vi "HandleObservationSync.vi"(8 "error in (no error)":errorcluster, 11 "S4ACS_GUI in":refnum<class "S4ACS_GUI.lvclass">) -> (0 "error out":errorcluster, 3 "S4ACS_GUI out":refnum<class "S4ACS_GUI.lvclass">)   [LabVIEW 2018, in "S4ACS_GUI.lvclass"]
uses:
  S4ACS_GUI.lvclass
  S4ACS_GUI.lvclass/S4ACS_GUI.ctl
  Instrument/Instrument.lvclass/Instrument.ctl
  Device/Optics/Optics.lvclass/Optics.ctl
  Server/Server.lvclass/Server.ctl
  Device/Optics/Opt_Selector/Opt_Selector.lvclass
  C:/Users/observer/Desktop/Sparc4GUI/SPARC4_GUI/Device/Optics/Optics.lvclass
  Acquisition/Acquisition.lvclass
  C:/Users/observer/Desktop/Sparc4GUI/SPARC4_GUI/Server/Server.lvclass
  SyncBox/Sync Box.lvclass
  Instrument/Instrument.lvclass
  StateMachine/State Machine.lvclass
  Trigger/Trigger.lvclass
  Channel/Channel.lvclass
  Device/Optics/Optics.lvclass
  Server/Server.lvclass
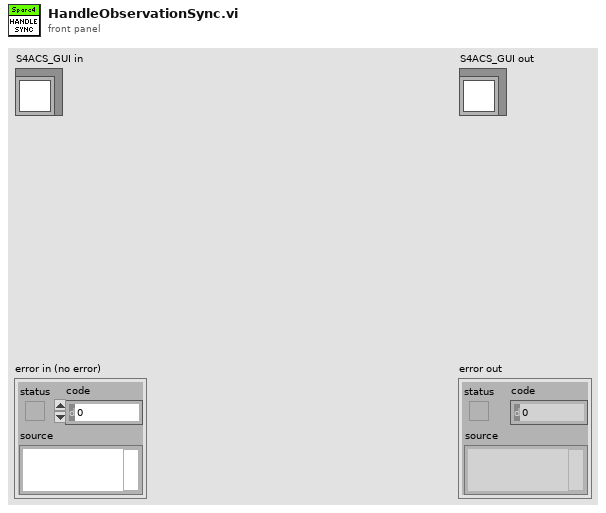
[diagram p1: front panel]
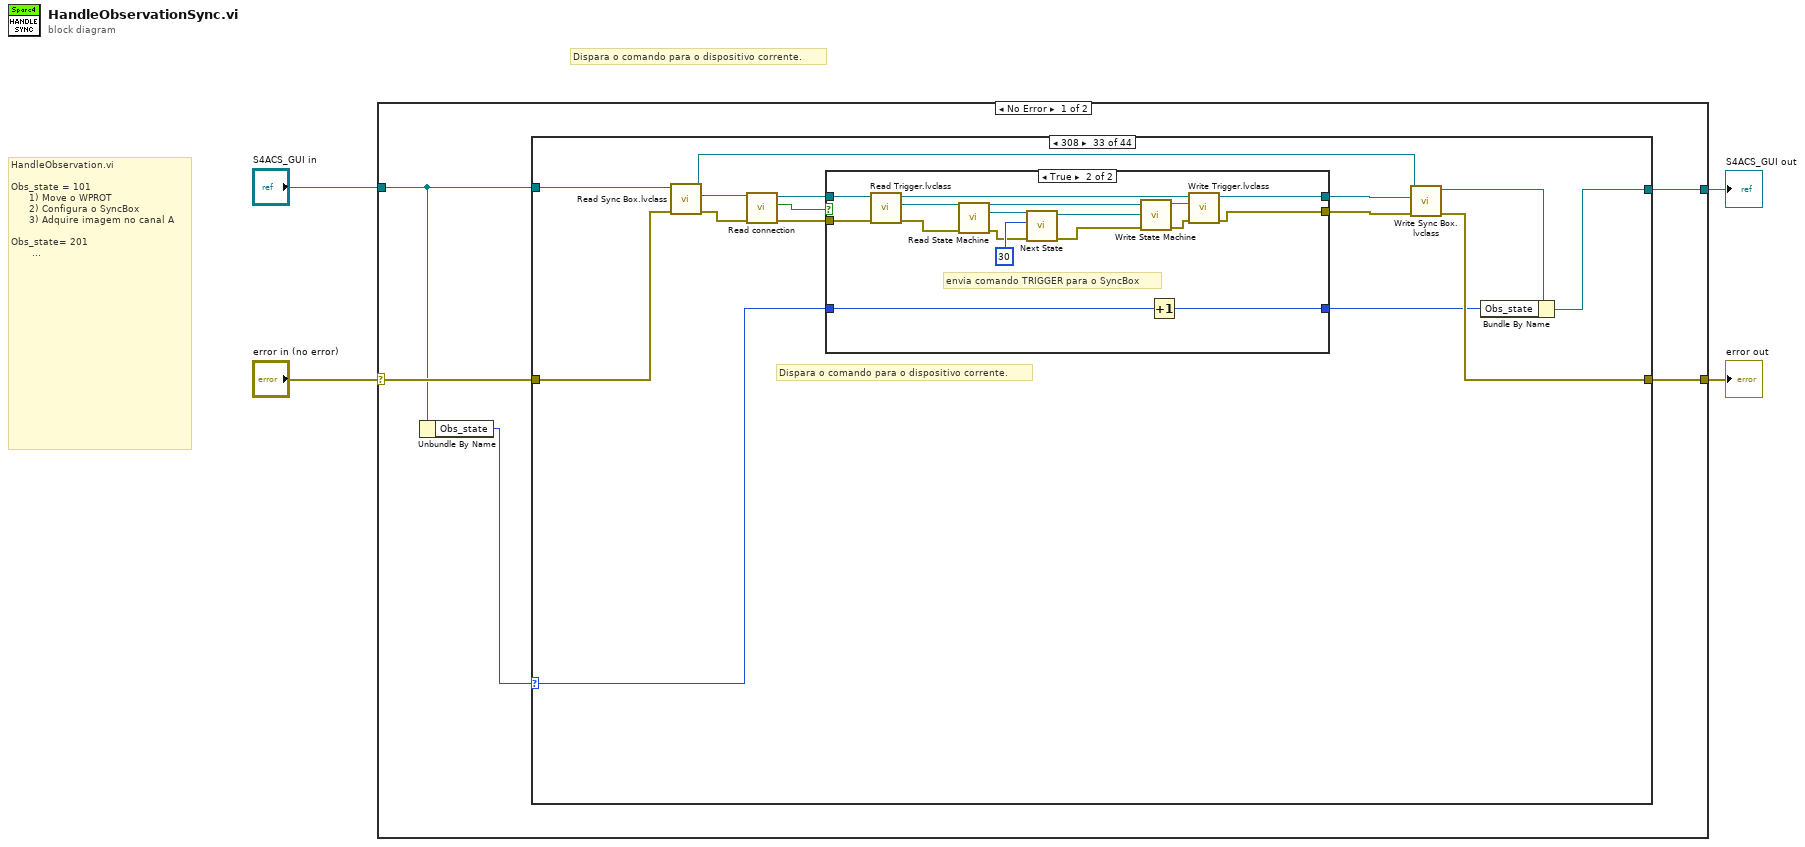
[diagram p0: block diagram]
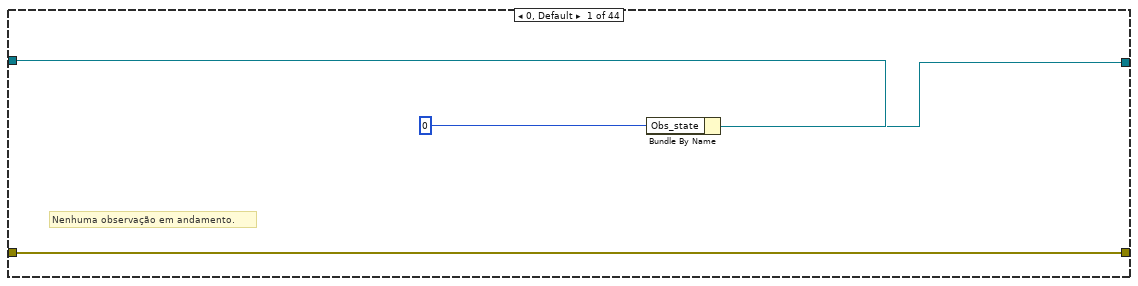
[diagram p2: hidden frame]
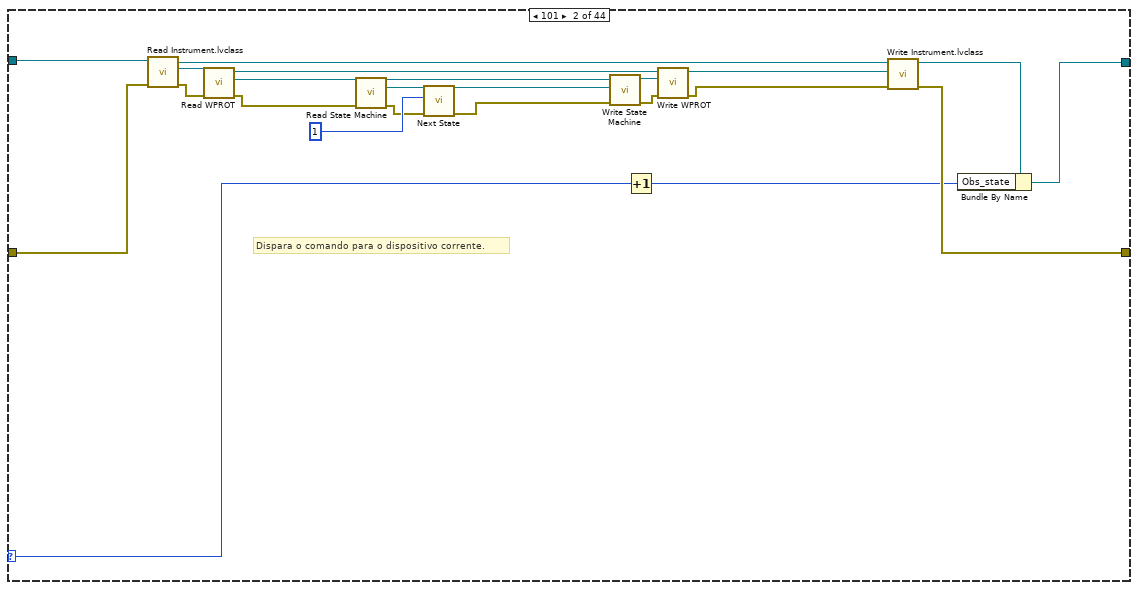
[diagram p3: hidden frame]
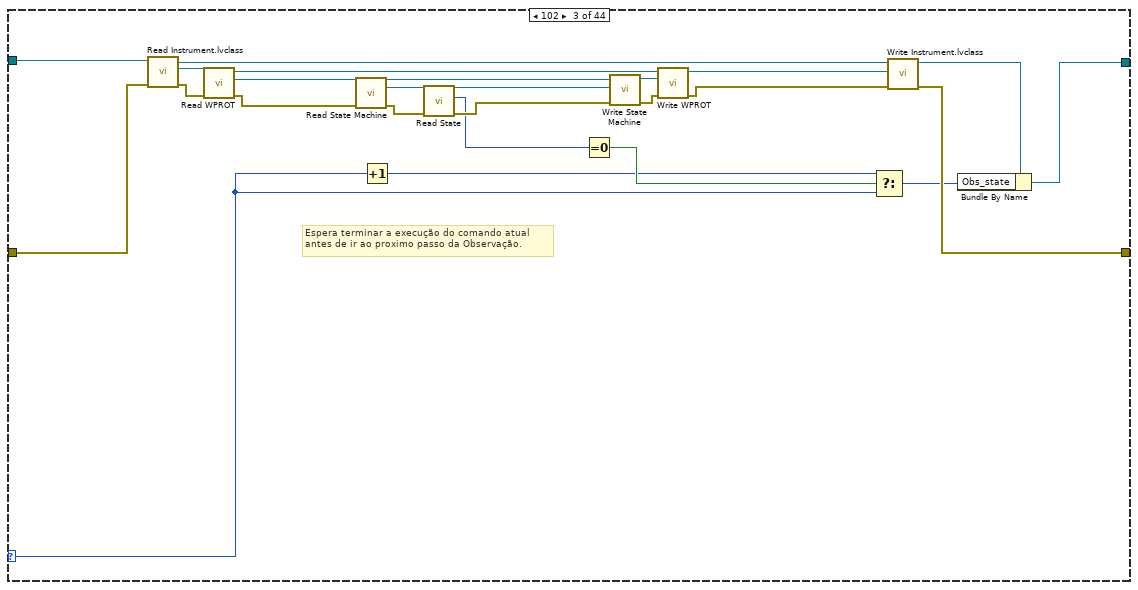
[diagram p4: hidden frame]
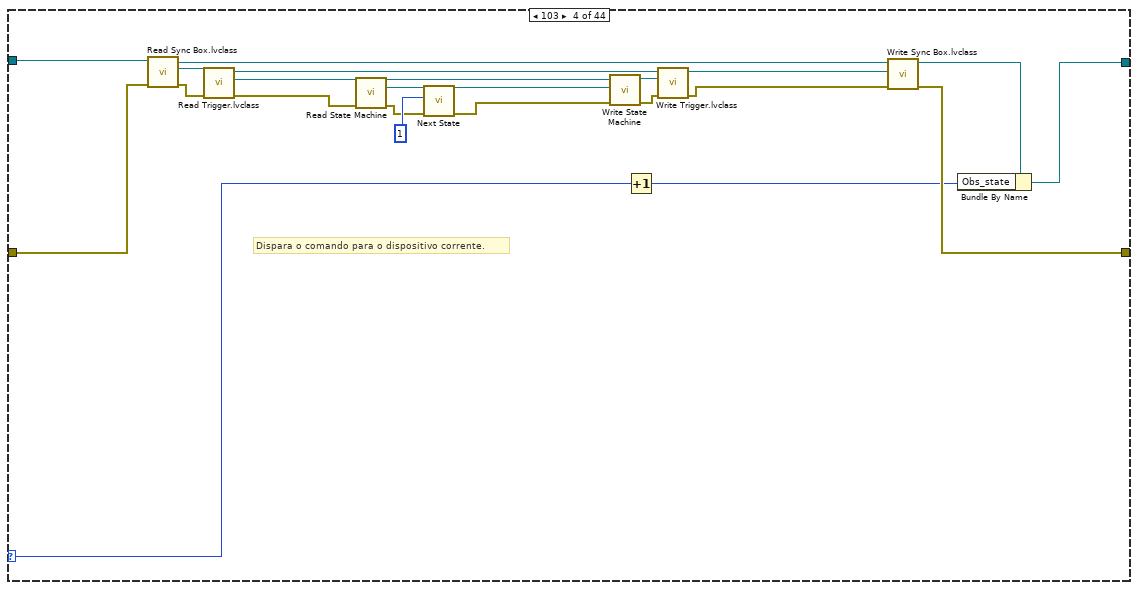
[diagram p5: hidden frame]
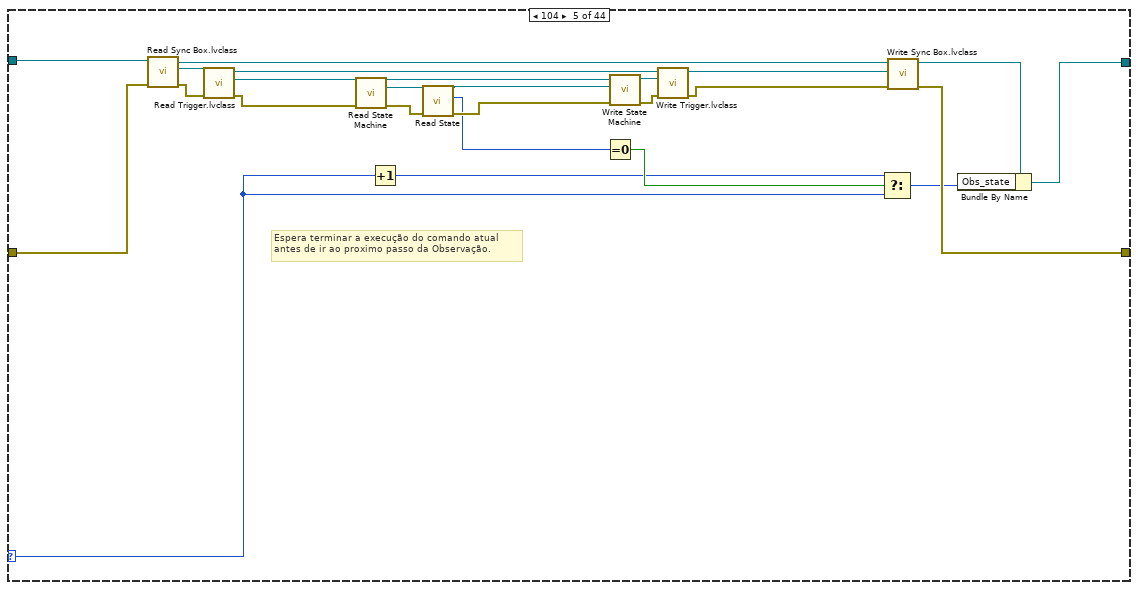
[diagram p6: hidden frame]
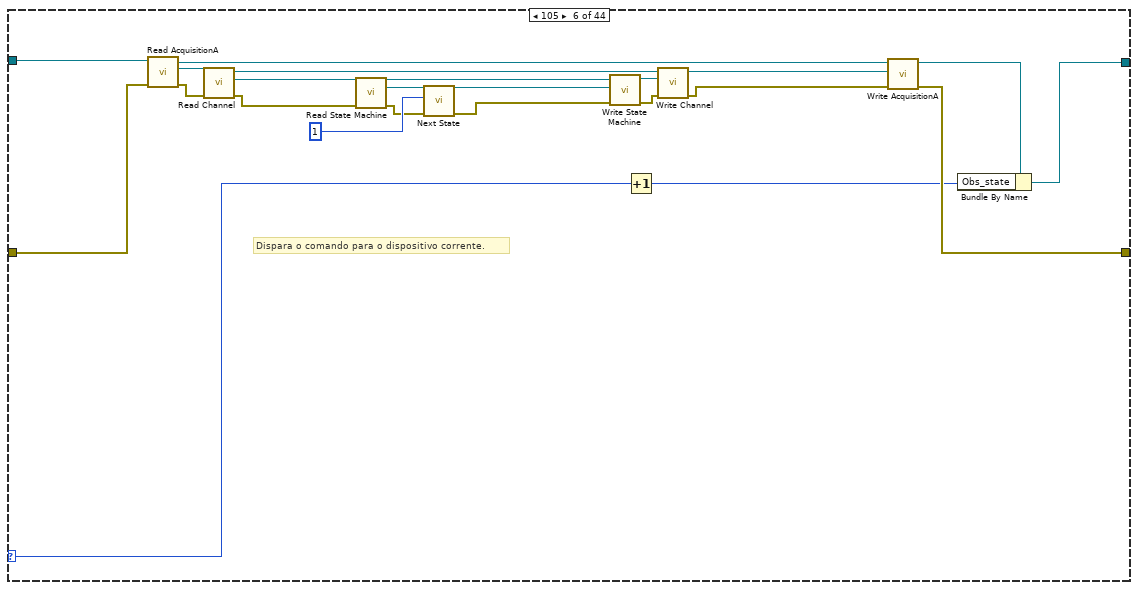
[diagram p7: hidden frame]
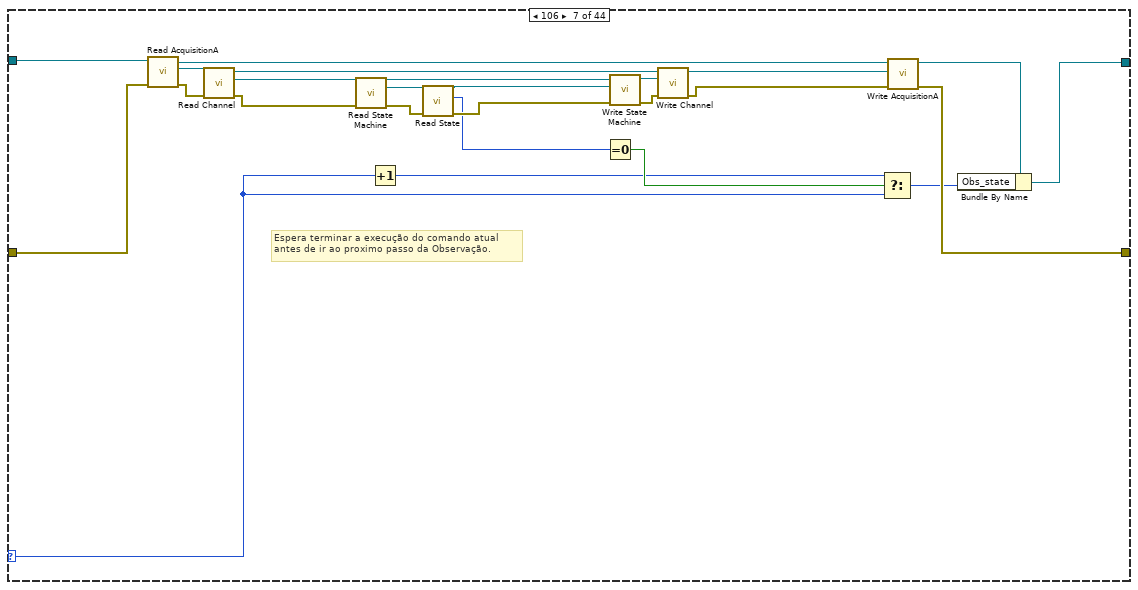
[diagram p8: hidden frame]
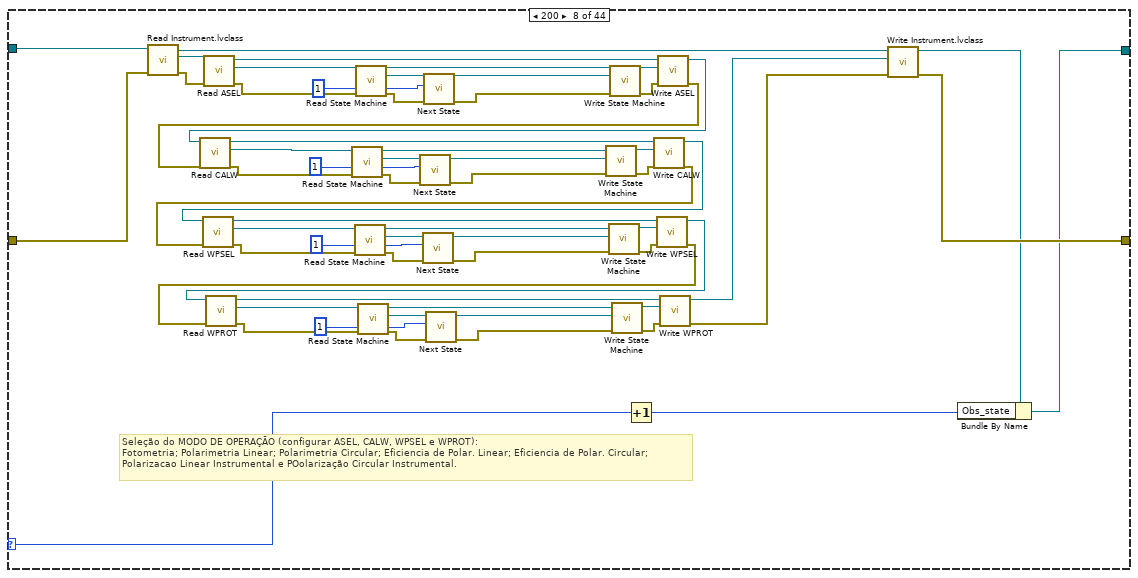
[diagram p9: hidden frame]
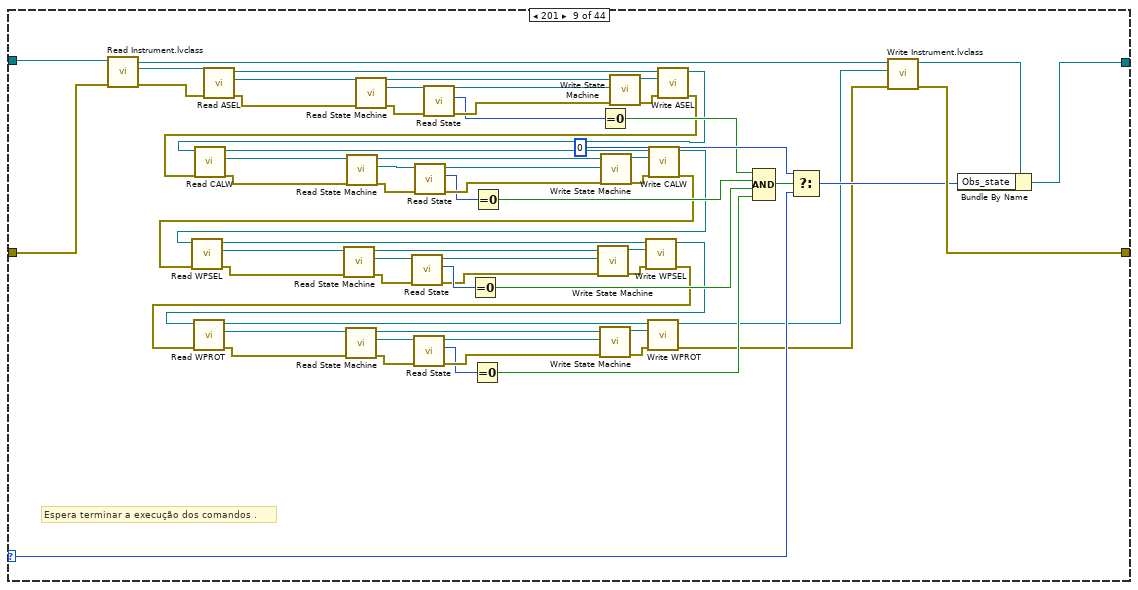
[diagram p10: hidden frame]
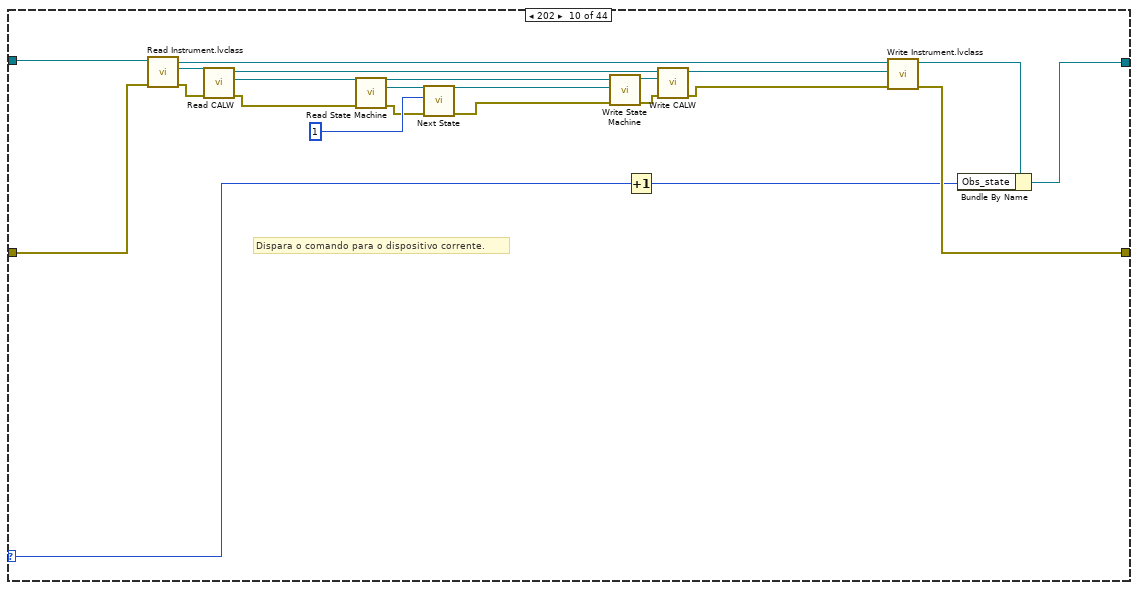
[diagram p11: hidden frame]
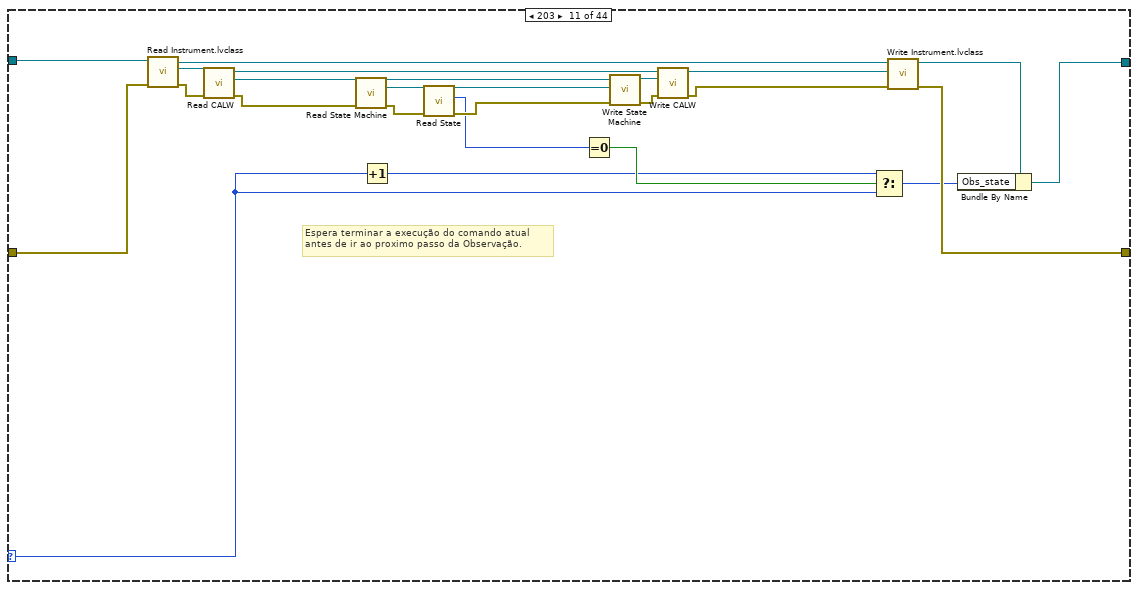
[diagram p12: hidden frame]
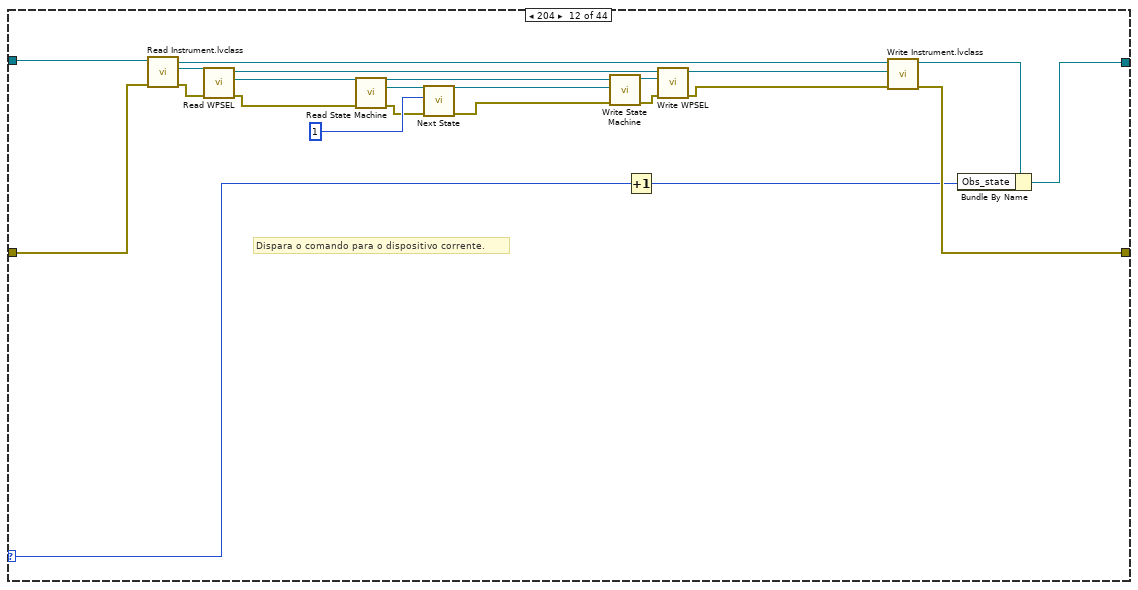
[diagram p13: hidden frame]
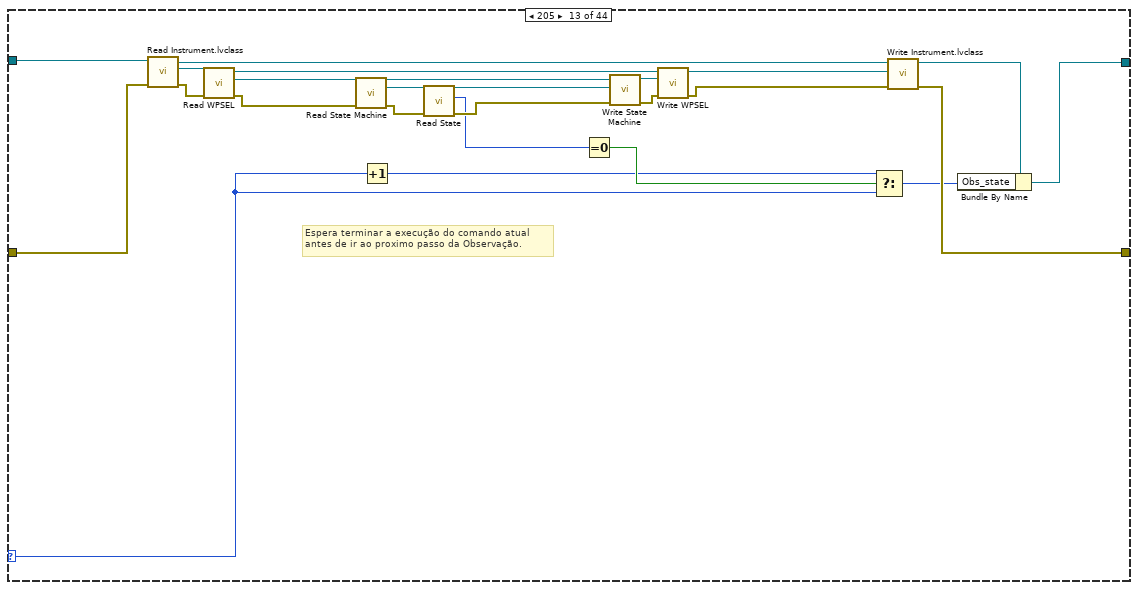
[diagram p14: hidden frame]
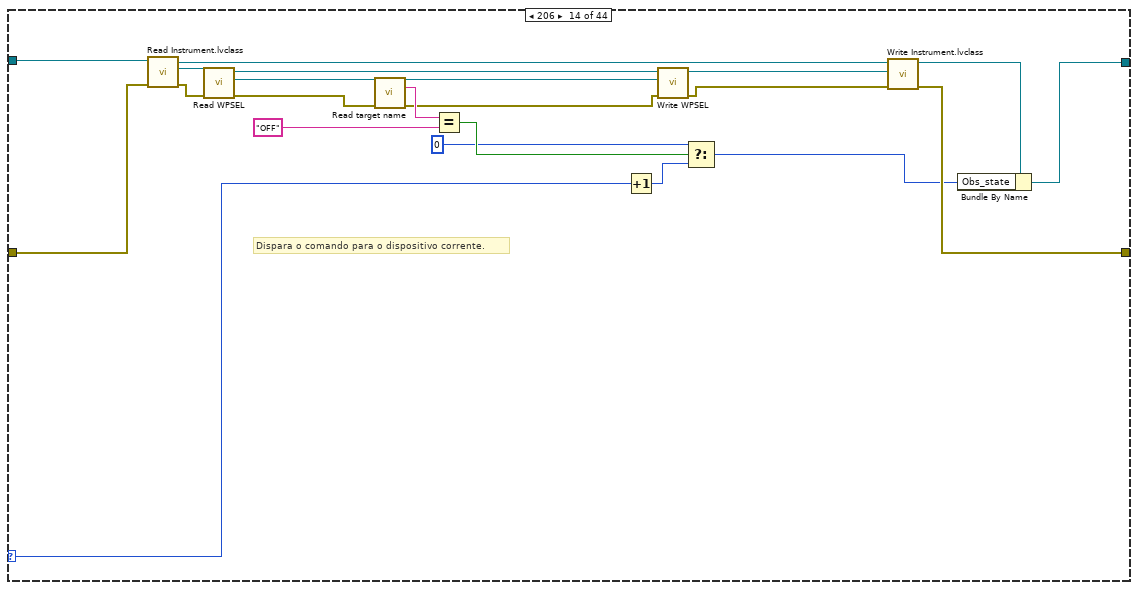
[diagram p15: hidden frame]
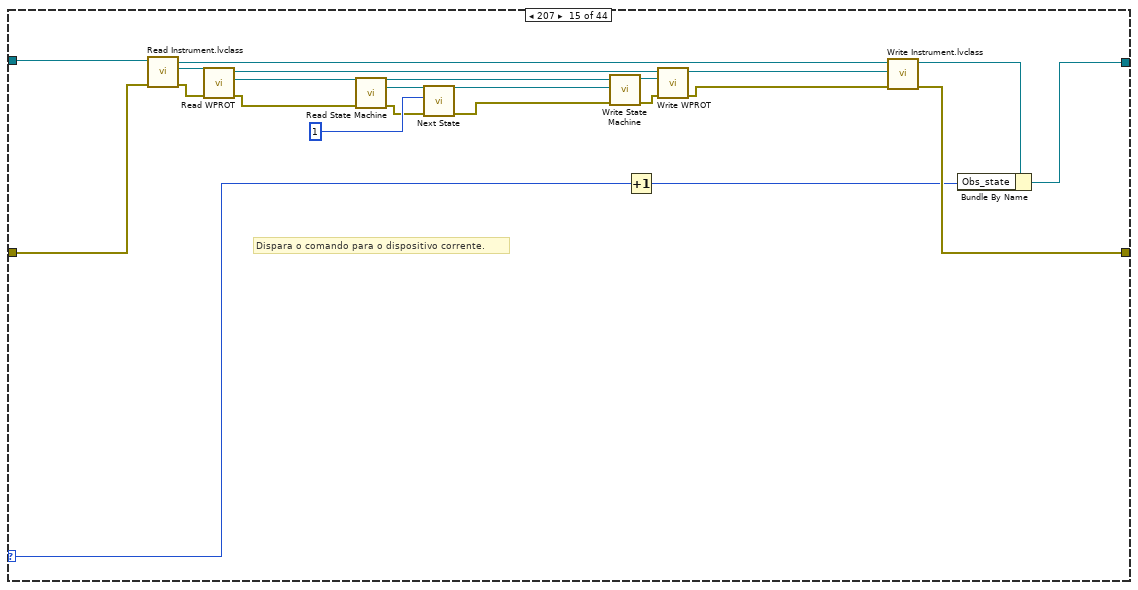
[diagram p16: hidden frame]
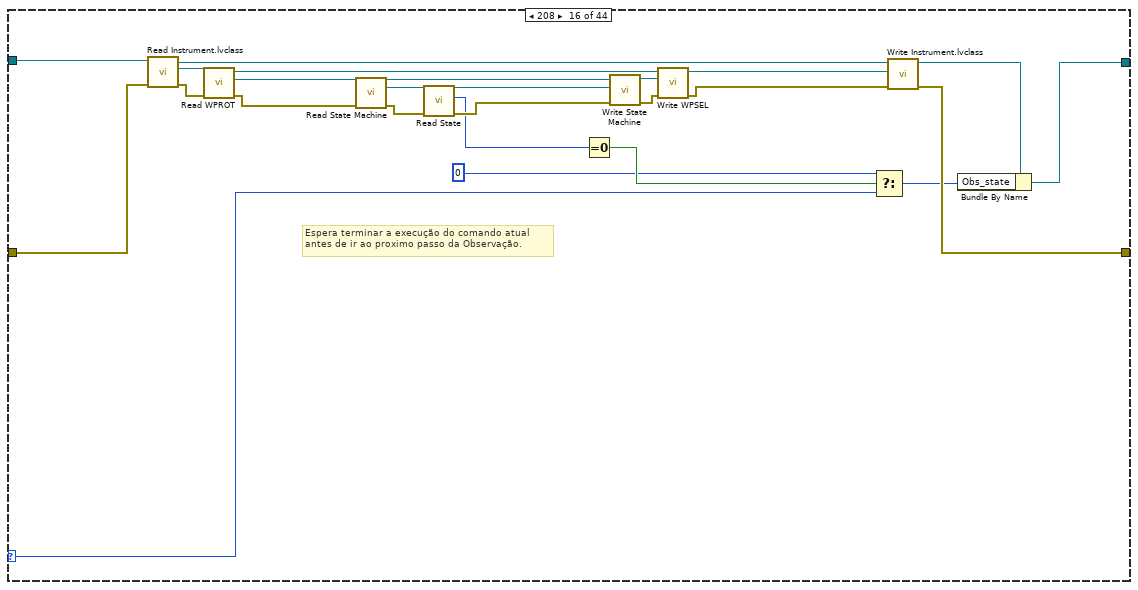
[diagram p17: hidden frame]
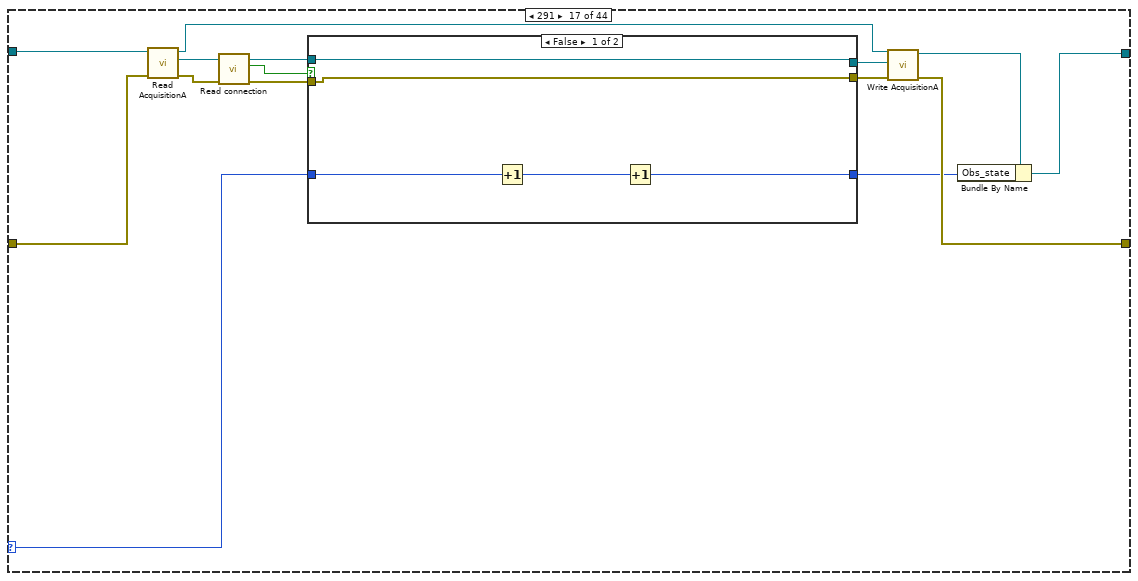
[diagram p18: hidden frame]
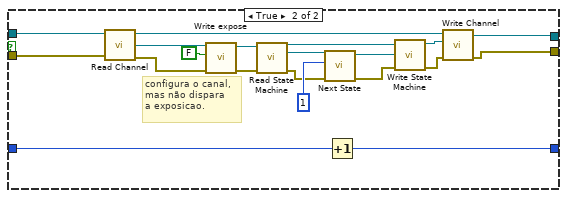
[diagram p19: hidden frame]
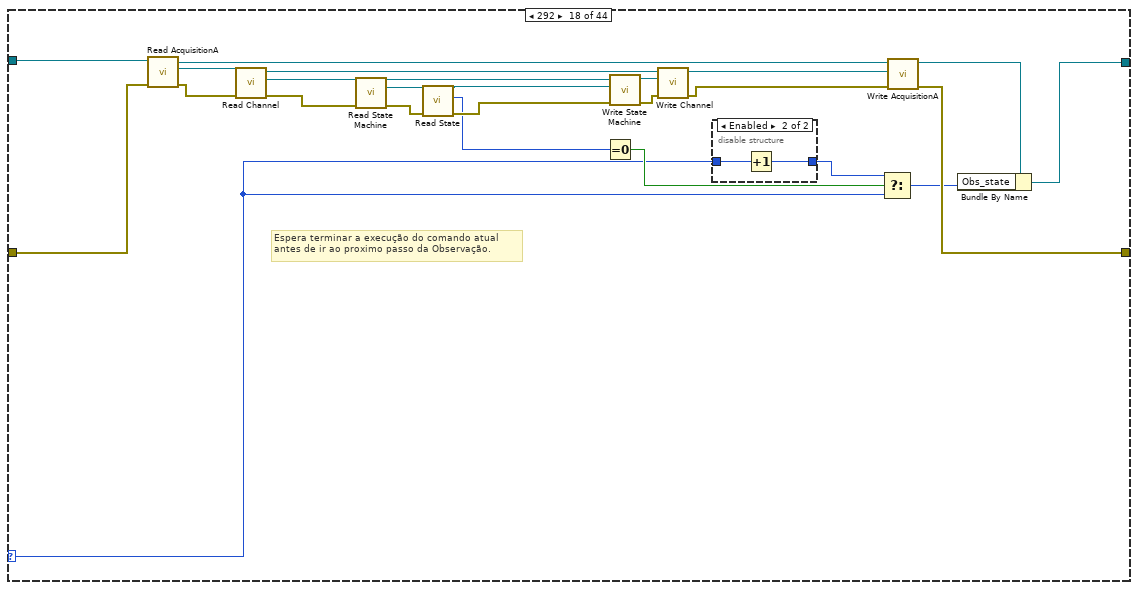
[diagram p20: hidden frame]
diagram:
  # "Dispara o comando para o dispositivo corrente."
  # "HandleObservation.vi\n\nObs_state = 101\n      1) Move o WPROT\n      2) Configura o SyncBox\n      3) Adquire imagem no canal A\n\nObs_state= 201\n       ..."
  n1 = case shown="No Error" "error in (no error)" {
    selector: "error in (no error)" -> [w8 w1585]
    tunnel: [w7 w1585] -> w3
    tunnel: [w9 w1584] -> w1
    tunnel: "S4ACS_GUI in" -> [w6 w1584]
    frame No Error {
      n2 = Unbundle By Name(w6) -> ("Obs_state"=w5:u32)
      n3 = case shown="308" w5 {
        selector: w5 -> [_ w16 w38 w64 w86 w112 w134 w202 w265 w290 w312 w338 w360 w395 w408 w430 w461 w494 w529 w563 w594 w628 w659 w693 _ w759 w805 w827 w858 w892 w955 w1041 w1077 w1108 w1187 _ w1232 w1272 w1340 w1422 w1459 w1543 _ _]
        tunnel: w6 -> [w12 w30 w55 w78 w103 w126 w151 w216 w283 w304 w329 w352 w377 w399 w422 w447 w465 w512 w533 w580 w598 w645 w663 w710 w727 w763 w820 w844 w862 w909 w957 w1058 w1081 w1125 w1205 w1225 w1242 w1289 w1299 w1432 w1476 w1556 w1576 w1583]
        tunnel: [w10 w14 w42 w62 w94 w110 w142 w200 w270 w288 w316 w336 w364 w394 w406 w434 w459 w503 w527 w571 w592 w636 w657 w701 w725 w757 w809 w835 w856 w900 w953 w1049 w1075 w1116 w1198 w1221 w1238 w1280 w1338 w1428 w1467 w1549 w1572 w1583] -> w9
        tunnel: w8 -> [w13 w29 w54 w77 w102 w125 w150 w215 w282 w303 w328 w351 w376 w398 w421 w446 w464 w511 w532 w579 w597 w644 w662 w709 w726 w762 w819 w843 w861 w908 w956 w1057 w1080 w1124 w1204 w1224 w1241 w1288 w1298 w1431 w1475 w1555 w1575 w1582]
        tunnel: [w13 w28 w53 w76 w101 w124 w149 w214 w281 w302 w327 w350 w375 w397 w420 w445 w463 w510 w531 w578 w596 w643 w661 w708 w717 w761 w818 w842 w860 w907 w937 w1056 w1079 w1123 w1132 w1223 w1240 w1287 w1296 w1430 w1474 w1485 w1574 w1582] -> w7
        frame 0, Default {
          # "Nenhuma observação em andamento."
          n4 = Bundle By Name(cluster=w12, "Obs_state"=u32 0) -> (w10:refnum<class "S4ACS_GUI.lvclass">)
        }
        frame 101 {
          # "Dispara o comando para o dispositivo corrente."
          n5 = call "Read Instrument.lvclass.vi"("error in (no error)"=w29, "S4ACS_GUI in"=w30) -> ("error out"=w35:errorcluster, "Instrument.lvclass"=w36:refnum<class "Instrument.lvclass">, "S4ACS_GUI out"=w32:refnum<class "S4ACS_GUI.lvclass">)  [unwired: 7 in]
          n6 = call "Read WPROT.vi"("error in (no error)"=w35, "Instrument in"=w36) -> ("error out"=w22:errorcluster, "Opt_Selector.lvclass"=w21:refnum<class "Opt_Selector.lvclass">, "Instrument out"=w34:refnum<class "Instrument.lvclass">)  [unwired: 7 in]
          n7 = call-dynamic "Read State Machine.vi"("error in (no error)"=w22, "Device in"=w21) -> ("error out"=w25:errorcluster, "State Machine.lvclass"=w27:refnum<class "State Machine.lvclass">, "Device out"=w19:refnum<class "Opt_Selector.lvclass">)  [unwired: 7 in]
          n8 = call "Next State.vi"("error in (no error)"=w25, "New_State"=1, "State Machine in"=w27) -> ("error out"=w24:errorcluster, "State Machine out"=w23:refnum<class "State Machine.lvclass">)  [unwired: 7 in]
          n9 = call-dynamic "Write State Machine.vi"("error in (no error)"=w24, "State Machine.lvclass"=w23, "Device in"=w19) -> ("error out"=w18:errorcluster, "Device out"=w20:refnum<class "Opt_Selector.lvclass">)  [unwired: 7 in]
          n10 = Increment(x=w16) -> (x+1=w15:u32)
          n11 = call "Write WPROT.vi"("error in (no error)"=w18, "Opt_Selector.lvclass"=w20, "Instrument in"=w34) -> ("error out"=w31:errorcluster, "Instrument out"=w33:refnum<class "Instrument.lvclass">)  [unwired: 7 in]
          n12 = call "Write Instrument.lvclass.vi"("error in (no error)"=w31, "Instrument.lvclass"=w33, "S4ACS_GUI in"=w32) -> ("error out"=w28:errorcluster, "S4ACS_GUI out"=w17:refnum<class "S4ACS_GUI.lvclass">)  [unwired: 7 in]
          n13 = Bundle By Name(cluster=w17, "Obs_state"=w15) -> (w14:refnum<class "S4ACS_GUI.lvclass">)
        }
        frame 102 {
          # "Espera terminar a execução do comando atual \nantes de ir ao proximo passo da Observação."
          n14 = call "Read Instrument.lvclass.vi"("error in (no error)"=w54, "S4ACS_GUI in"=w55) -> ("error out"=w60:errorcluster, "Instrument.lvclass"=w61:refnum<class "Instrument.lvclass">, "S4ACS_GUI out"=w57:refnum<class "S4ACS_GUI.lvclass">)  [unwired: 7 in]
          n15 = call "Read WPROT.vi"("error in (no error)"=w60, "Instrument in"=w61) -> ("error out"=w48:errorcluster, "Opt_Selector.lvclass"=w47:refnum<class "Opt_Selector.lvclass">, "Instrument out"=w59:refnum<class "Instrument.lvclass">)  [unwired: 7 in]
          n16 = call-dynamic "Read State Machine.vi"("error in (no error)"=w48, "Device in"=w47) -> ("error out"=w51:errorcluster, "State Machine.lvclass"=w52:refnum<class "State Machine.lvclass">, "Device out"=w45:refnum<class "Opt_Selector.lvclass">)  [unwired: 7 in]
          n17 = Increment(x=w38) -> (x+1=w37:u32)
          n18 = call-dynamic "Read State.vi"("error in (no error)"=w51, "State Machine in"=w52) -> ("error out"=w50:errorcluster, "State"=w40:i32, "State Machine out"=w49:refnum<class "State Machine.lvclass">)  [unwired: 7 in]
          n19 = Equal To 0?(x=w40) -> (x = 0?=w41:bool)
          n20 = call-dynamic "Write State Machine.vi"("error in (no error)"=w50, "State Machine.lvclass"=w49, "Device in"=w45) -> ("error out"=w44:errorcluster, "Device out"=w46:refnum<class "Opt_Selector.lvclass">)  [unwired: 7 in]
          n21 = call "Write WPROT.vi"("error in (no error)"=w44, "Opt_Selector.lvclass"=w46, "Instrument in"=w59) -> ("error out"=w56:errorcluster, "Instrument out"=w58:refnum<class "Instrument.lvclass">)  [unwired: 7 in]
          n22 = Select(t=w37, s=w41, f=w38) -> (s? t:f=w39:u32)
          n23 = call "Write Instrument.lvclass.vi"("error in (no error)"=w56, "Instrument.lvclass"=w58, "S4ACS_GUI in"=w57) -> ("error out"=w53:errorcluster, "S4ACS_GUI out"=w43:refnum<class "S4ACS_GUI.lvclass">)  [unwired: 7 in]
          n24 = Bundle By Name(cluster=w43, "Obs_state"=w39) -> (w42:refnum<class "S4ACS_GUI.lvclass">)
        }
        frame 103 {
          # "Dispara o comando para o dispositivo corrente."
          n25 = call-dynamic "Read Sync Box.lvclass.vi"("error in (no error)"=w77, "SPARC4_AC in"=w78) -> ("error out"=w83:errorcluster, "Sync Box.lvclass"=w84:refnum<class "Sync Box.lvclass">, "SPARC4_AC out"=w80:refnum<class "S4ACS_GUI.lvclass">)  [unwired: 7 in]
          n26 = call-dynamic "Read Trigger.lvclass.vi"("error in (no error)"=w83, "Sync Box in"=w84) -> ("error out"=w70:errorcluster, "Trigger.lvclass"=w69:refnum<class "Trigger.lvclass">, "Sync Box out"=w82:refnum<class "Sync Box.lvclass">)  [unwired: 7 in]
          n27 = call-dynamic "Read State Machine.vi"("error in (no error)"=w70, "Device in"=w69) -> ("error out"=w73:errorcluster, "State Machine.lvclass"=w75:refnum<class "State Machine.lvclass">, "Device out"=w67:refnum<class "Trigger.lvclass">)  [unwired: 7 in]
          n28 = call "Next State.vi"("error in (no error)"=w73, "New_State"=1, "State Machine in"=w75) -> ("error out"=w72:errorcluster, "State Machine out"=w71:refnum<class "State Machine.lvclass">)  [unwired: 7 in]
          n29 = call-dynamic "Write State Machine.vi"("error in (no error)"=w72, "State Machine.lvclass"=w71, "Device in"=w67) -> ("error out"=w66:errorcluster, "Device out"=w68:refnum<class "Trigger.lvclass">)  [unwired: 7 in]
          n30 = Increment(x=w64) -> (x+1=w63:u32)
          n31 = call-dynamic "Write Trigger.lvclass.vi"("error in (no error)"=w66, "Trigger.lvclass"=w68, "Sync Box in"=w82) -> ("error out"=w79:errorcluster, "Sync Box out"=w81:refnum<class "Sync Box.lvclass">)  [unwired: 7 in]
          n32 = call-dynamic "Write Sync Box.lvclass.vi"("error in (no error)"=w79, "Sync Box.lvclass"=w81, "SPARC4_AC in"=w80) -> ("error out"=w76:errorcluster, "SPARC4_AC out"=w65:refnum<class "S4ACS_GUI.lvclass">)  [unwired: 7 in]
          n33 = Bundle By Name(cluster=w65, "Obs_state"=w63) -> (w62:refnum<class "S4ACS_GUI.lvclass">)
        }
        frame 104 {
          # "Espera terminar a execução do comando atual \nantes de ir ao proximo passo da Observação."
          n34 = call-dynamic "Read Sync Box.lvclass.vi"("error in (no error)"=w102, "SPARC4_AC in"=w103) -> ("error out"=w108:errorcluster, "Sync Box.lvclass"=w109:refnum<class "Sync Box.lvclass">, "SPARC4_AC out"=w105:refnum<class "S4ACS_GUI.lvclass">)  [unwired: 7 in]
          n35 = call-dynamic "Read Trigger.lvclass.vi"("error in (no error)"=w108, "Sync Box in"=w109) -> ("error out"=w100:errorcluster, "Trigger.lvclass"=w99:refnum<class "Trigger.lvclass">, "Sync Box out"=w107:refnum<class "Sync Box.lvclass">)  [unwired: 7 in]
          n36 = call-dynamic "Read State Machine.vi"("error in (no error)"=w100, "Device in"=w99) -> ("error out"=w91:errorcluster, "State Machine.lvclass"=w93:refnum<class "State Machine.lvclass">, "Device out"=w97:refnum<class "Trigger.lvclass">)  [unwired: 7 in]
          n37 = Increment(x=w86) -> (x+1=w88:u32)
          n38 = call-dynamic "Read State.vi"("error in (no error)"=w91, "State Machine in"=w93) -> ("error out"=w90:errorcluster, "State"=w85:i32, "State Machine out"=w92:refnum<class "State Machine.lvclass">)  [unwired: 7 in]
          n39 = Equal To 0?(x=w85) -> (x = 0?=w89:bool)
          n40 = call-dynamic "Write State Machine.vi"("error in (no error)"=w90, "State Machine.lvclass"=w92, "Device in"=w97) -> ("error out"=w96:errorcluster, "Device out"=w98:refnum<class "Trigger.lvclass">)  [unwired: 7 in]
          n41 = call-dynamic "Write Trigger.lvclass.vi"("error in (no error)"=w96, "Trigger.lvclass"=w98, "Sync Box in"=w107) -> ("error out"=w104:errorcluster, "Sync Box out"=w106:refnum<class "Sync Box.lvclass">)  [unwired: 7 in]
          n42 = Select(t=w88, s=w89, f=w86) -> (s? t:f=w87:u32)
          n43 = call-dynamic "Write Sync Box.lvclass.vi"("error in (no error)"=w104, "Sync Box.lvclass"=w106, "SPARC4_AC in"=w105) -> ("error out"=w101:errorcluster, "SPARC4_AC out"=w95:refnum<class "S4ACS_GUI.lvclass">)  [unwired: 7 in]
          n44 = Bundle By Name(cluster=w95, "Obs_state"=w87) -> (w94:refnum<class "S4ACS_GUI.lvclass">)
        }
        frame 105 {
          # "Dispara o comando para o dispositivo corrente."
          n45 = call-dynamic "Read AcquisitionA.vi"("error in (no error)"=w125, "S4ACS_GUI in"=w126) -> ("error out"=w131:errorcluster, "Acquisition.lvclass"=w132:refnum<class "Acquisition.lvclass">, "S4ACS_GUI out"=w128:refnum<class "S4ACS_GUI.lvclass">)  [unwired: 7 in]
          n46 = call-dynamic "Read Channel.vi"("error in (no error)"=w131, "Acquisition in"=w132) -> ("error out"=w118:errorcluster, "Channel.lvclass"=w117:refnum<class "Channel.lvclass">, "Acquisition out"=w130:refnum<class "Acquisition.lvclass">)  [unwired: 7 in]
          n47 = call-dynamic "Read State Machine.vi"("error in (no error)"=w118, "Device in"=w117) -> ("error out"=w121:errorcluster, "State Machine.lvclass"=w123:refnum<class "State Machine.lvclass">, "Device out"=w115:refnum<class "Channel.lvclass">)  [unwired: 7 in]
          n48 = call "Next State.vi"("error in (no error)"=w121, "New_State"=1, "State Machine in"=w123) -> ("error out"=w120:errorcluster, "State Machine out"=w119:refnum<class "State Machine.lvclass">)  [unwired: 7 in]
          n49 = call-dynamic "Write State Machine.vi"("error in (no error)"=w120, "State Machine.lvclass"=w119, "Device in"=w115) -> ("error out"=w114:errorcluster, "Device out"=w116:refnum<class "Channel.lvclass">)  [unwired: 7 in]
          n50 = Increment(x=w112) -> (x+1=w111:u32)
          n51 = call-dynamic "Write Channel.vi"("error in (no error)"=w114, "Channel.lvclass"=w116, "Acquisition in"=w130) -> ("error out"=w127:errorcluster, "Acquisition out"=w129:refnum<class "Acquisition.lvclass">)  [unwired: 7 in]
          n52 = call-dynamic "Write AcquisitionA.vi"("error in (no error)"=w127, "Acquisition.lvclass"=w129, "S4ACS_GUI in"=w128) -> ("error out"=w124:errorcluster, "S4ACS_GUI out"=w113:refnum<class "S4ACS_GUI.lvclass">)  [unwired: 7 in]
          n53 = Bundle By Name(cluster=w113, "Obs_state"=w111) -> (w110:refnum<class "S4ACS_GUI.lvclass">)
        }
        frame 106 {
          # "Espera terminar a execução do comando atual \nantes de ir ao proximo passo da Observação."
          n54 = call-dynamic "Read AcquisitionA.vi"("error in (no error)"=w150, "S4ACS_GUI in"=w151) -> ("error out"=w156:errorcluster, "Acquisition.lvclass"=w157:refnum<class "Acquisition.lvclass">, "S4ACS_GUI out"=w153:refnum<class "S4ACS_GUI.lvclass">)  [unwired: 7 in]
          n55 = call-dynamic "Read Channel.vi"("error in (no error)"=w156, "Acquisition in"=w157) -> ("error out"=w148:errorcluster, "Channel.lvclass"=w147:refnum<class "Channel.lvclass">, "Acquisition out"=w155:refnum<class "Acquisition.lvclass">)  [unwired: 7 in]
          n56 = call-dynamic "Read State Machine.vi"("error in (no error)"=w148, "Device in"=w147) -> ("error out"=w139:errorcluster, "State Machine.lvclass"=w141:refnum<class "State Machine.lvclass">, "Device out"=w145:refnum<class "Channel.lvclass">)  [unwired: 7 in]
          n57 = Increment(x=w134) -> (x+1=w136:u32)
          n58 = call-dynamic "Read State.vi"("error in (no error)"=w139, "State Machine in"=w141) -> ("error out"=w138:errorcluster, "State"=w133:i32, "State Machine out"=w140:refnum<class "State Machine.lvclass">)  [unwired: 7 in]
          n59 = Equal To 0?(x=w133) -> (x = 0?=w137:bool)
          n60 = call-dynamic "Write State Machine.vi"("error in (no error)"=w138, "State Machine.lvclass"=w140, "Device in"=w145) -> ("error out"=w144:errorcluster, "Device out"=w146:refnum<class "Channel.lvclass">)  [unwired: 7 in]
          n61 = call-dynamic "Write Channel.vi"("error in (no error)"=w144, "Channel.lvclass"=w146, "Acquisition in"=w155) -> ("error out"=w152:errorcluster, "Acquisition out"=w154:refnum<class "Acquisition.lvclass">)  [unwired: 7 in]
          n62 = Select(t=w136, s=w137, f=w134) -> (s? t:f=w135:u32)
          n63 = call-dynamic "Write AcquisitionA.vi"("error in (no error)"=w152, "Acquisition.lvclass"=w154, "S4ACS_GUI in"=w153) -> ("error out"=w149:errorcluster, "S4ACS_GUI out"=w143:refnum<class "S4ACS_GUI.lvclass">)  [unwired: 7 in]
          n64 = Bundle By Name(cluster=w143, "Obs_state"=w135) -> (w142:refnum<class "S4ACS_GUI.lvclass">)
        }
        frame 200 {
          # "Seleção do MODO DE OPERAÇÃO (configurar ASEL, CALW, WPSEL e WPROT): \nFotometria; Polarimetria Linear; Polarimetria Circular; Eficiencia de Polar. Linear; Eficiencia de Polar. Circular;\nPolarizacao Linear Instrumental e POolarização Circular Instrumental."
          n65 = call "Read Instrument.lvclass.vi"("error in (no error)"=w215, "S4ACS_GUI in"=w216) -> ("error out"=w219:errorcluster, "Instrument.lvclass"=w179:refnum<class "Instrument.lvclass">, "S4ACS_GUI out"=w217:refnum<class "S4ACS_GUI.lvclass">)  [unwired: 7 in]
          n66 = call "Read ASEL.vi"("error in (no error)"=w219, "Instrument in"=w179) -> ("error out"=w208:errorcluster, "Opt_Selector.lvclass"=w207:refnum<class "Opt_Selector.lvclass">, "Instrument out"=w218:refnum<class "Instrument.lvclass">)  [unwired: 7 in]
          n67 = call-dynamic "Read State Machine.vi"("error in (no error)"=w208, "Device in"=w207) -> ("error out"=w211:errorcluster, "State Machine.lvclass"=w213:refnum<class "State Machine.lvclass">, "Device out"=w205:refnum<class "Opt_Selector.lvclass">)  [unwired: 7 in]
          n68 = call "Next State.vi"("error in (no error)"=w211, "New_State"=1, "State Machine in"=w213) -> ("error out"=w210:errorcluster, "State Machine out"=w209:refnum<class "State Machine.lvclass">)  [unwired: 7 in]
          n69 = call-dynamic "Write State Machine.vi"("error in (no error)"=w210, "State Machine.lvclass"=w209, "Device in"=w205) -> ("error out"=w204:errorcluster, "Device out"=w206:refnum<class "Opt_Selector.lvclass">)  [unwired: 7 in]
          n70 = Increment(x=w202) -> (x+1=w201:u32)
          n71 = call "Write ASEL.vi"("error in (no error)"=w204, "Opt_Selector.lvclass"=w206, "Instrument in"=w218) -> ("error out"=w160:errorcluster, "Instrument out"=w178:refnum<class "Instrument.lvclass">)  [unwired: 7 in]
          n72 = call "Read CALW.vi"("error in (no error)"=w160, "Instrument in"=w178) -> ("error out"=w195:errorcluster, "Opt_Selector.lvclass"=w196:refnum<class "Opt_Selector.lvclass">, "Instrument out"=w177:refnum<class "Instrument.lvclass">)  [unwired: 7 in]
          n73 = call-dynamic "Read State Machine.vi"("error in (no error)"=w195, "Device in"=w196) -> ("error out"=w192:errorcluster, "State Machine.lvclass"=w190:refnum<class "State Machine.lvclass">, "Device out"=w198:refnum<class "Opt_Selector.lvclass">)  [unwired: 7 in]
          n74 = call "Next State.vi"("error in (no error)"=w192, "New_State"=1, "State Machine in"=w190) -> ("error out"=w193:errorcluster, "State Machine out"=w194:refnum<class "State Machine.lvclass">)  [unwired: 7 in]
          n75 = call-dynamic "Write State Machine.vi"("error in (no error)"=w193, "State Machine.lvclass"=w194, "Device in"=w198) -> ("error out"=w199:errorcluster, "Device out"=w197:refnum<class "Opt_Selector.lvclass">)  [unwired: 7 in]
          n76 = call "Write CALW.vi"("error in (no error)"=w199, "Opt_Selector.lvclass"=w197, "Instrument in"=w177) -> ("error out"=w159:errorcluster, "Instrument out"=w176:refnum<class "Instrument.lvclass">)  [unwired: 7 in]
          n77 = call "Read WPSEL.vi"("error in (no error)"=w159, "Instrument in"=w176) -> ("error out"=w184:errorcluster, "Opt_Selector.lvclass"=w183:refnum<class "Opt_Selector.lvclass">, "Instrument out"=w175:refnum<class "Instrument.lvclass">)  [unwired: 7 in]
          n78 = call-dynamic "Read State Machine.vi"("error in (no error)"=w184, "Device in"=w183) -> ("error out"=w187:errorcluster, "State Machine.lvclass"=w189:refnum<class "State Machine.lvclass">, "Device out"=w181:refnum<class "Opt_Selector.lvclass">)  [unwired: 7 in]
          n79 = call "Next State.vi"("error in (no error)"=w187, "New_State"=1, "State Machine in"=w189) -> ("error out"=w186:errorcluster, "State Machine out"=w185:refnum<class "State Machine.lvclass">)  [unwired: 7 in]
          n80 = call-dynamic "Write State Machine.vi"("error in (no error)"=w186, "State Machine.lvclass"=w185, "Device in"=w181) -> ("error out"=w180:errorcluster, "Device out"=w182:refnum<class "Opt_Selector.lvclass">)  [unwired: 7 in]
          n81 = call "Write WPSEL.vi"("error in (no error)"=w180, "Opt_Selector.lvclass"=w182, "Instrument in"=w175) -> ("error out"=w158:errorcluster, "Instrument out"=w164:refnum<class "Instrument.lvclass">)  [unwired: 7 in]
          n82 = call "Read WPROT.vi"("error in (no error)"=w158, "Instrument in"=w164) -> ("error out"=w170:errorcluster, "Opt_Selector.lvclass"=w171:refnum<class "Opt_Selector.lvclass">, "Instrument out"=w163:refnum<class "Instrument.lvclass">)  [unwired: 7 in]
          n83 = call-dynamic "Read State Machine.vi"("error in (no error)"=w170, "Device in"=w171) -> ("error out"=w167:errorcluster, "State Machine.lvclass"=w165:refnum<class "State Machine.lvclass">, "Device out"=w173:refnum<class "Opt_Selector.lvclass">)  [unwired: 7 in]
          n84 = call "Next State.vi"("error in (no error)"=w167, "New_State"=1, "State Machine in"=w165) -> ("error out"=w168:errorcluster, "State Machine out"=w169:refnum<class "State Machine.lvclass">)  [unwired: 7 in]
          n85 = call-dynamic "Write State Machine.vi"("error in (no error)"=w168, "State Machine.lvclass"=w169, "Device in"=w173) -> ("error out"=w174:errorcluster, "Device out"=w172:refnum<class "Opt_Selector.lvclass">)  [unwired: 7 in]
          n86 = call "Write WPROT.vi"("error in (no error)"=w174, "Opt_Selector.lvclass"=w172, "Instrument in"=w163) -> ("error out"=w161:errorcluster, "Instrument out"=w162:refnum<class "Instrument.lvclass">)  [unwired: 7 in]
          n87 = call "Write Instrument.lvclass.vi"("error in (no error)"=w161, "Instrument.lvclass"=w162, "S4ACS_GUI in"=w217) -> ("error out"=w214:errorcluster, "S4ACS_GUI out"=w203:refnum<class "S4ACS_GUI.lvclass">)  [unwired: 7 in]
          n88 = Bundle By Name(cluster=w203, "Obs_state"=w201) -> (w200:refnum<class "S4ACS_GUI.lvclass">)
        }
        frame 201 {
          # "Espera terminar a execução dos comandos ."
          n89 = call "Read Instrument.lvclass.vi"("error in (no error)"=w282, "S4ACS_GUI in"=w283) -> ("error out"=w286:errorcluster, "Instrument.lvclass"=w287:refnum<class "Instrument.lvclass">, "S4ACS_GUI out"=w284:refnum<class "S4ACS_GUI.lvclass">)  [unwired: 7 in]
          n90 = call "Read ASEL.vi"("error in (no error)"=w286, "Instrument in"=w287) -> ("error out"=w276:errorcluster, "Opt_Selector.lvclass"=w275:refnum<class "Opt_Selector.lvclass">, "Instrument out"=w285:refnum<class "Instrument.lvclass">)  [unwired: 7 in]
          n91 = call-dynamic "Read State Machine.vi"("error in (no error)"=w276, "Device in"=w275) -> ("error out"=w279:errorcluster, "State Machine.lvclass"=w280:refnum<class "State Machine.lvclass">, "Device out"=w273:refnum<class "Opt_Selector.lvclass">)  [unwired: 7 in]
          n92 = call-dynamic "Read State.vi"("error in (no error)"=w279, "State Machine in"=w280) -> ("error out"=w278:errorcluster, "State"=w269:i32, "State Machine out"=w277:refnum<class "State Machine.lvclass">)  [unwired: 7 in]
          n93 = Equal To 0?(x=w269) -> (x = 0?=w264:bool)
          n94 = call-dynamic "Write State Machine.vi"("error in (no error)"=w278, "State Machine.lvclass"=w277, "Device in"=w273) -> ("error out"=w272:errorcluster, "Device out"=w274:refnum<class "Opt_Selector.lvclass">)  [unwired: 7 in]
          n95 = call "Write ASEL.vi"("error in (no error)"=w272, "Opt_Selector.lvclass"=w274, "Instrument in"=w285) -> ("error out"=w226:errorcluster, "Instrument out"=w227:refnum<class "Instrument.lvclass">)  [unwired: 7 in]
          n96 = call "Read CALW.vi"("error in (no error)"=w226, "Instrument in"=w227) -> ("error out"=w259:errorcluster, "Opt_Selector.lvclass"=w260:refnum<class "Opt_Selector.lvclass">, "Instrument out"=w230:refnum<class "Instrument.lvclass">)  [unwired: 7 in]
          n97 = call-dynamic "Read State Machine.vi"("error in (no error)"=w259, "Device in"=w260) -> ("error out"=w256:errorcluster, "State Machine.lvclass"=w255:refnum<class "State Machine.lvclass">, "Device out"=w262:refnum<class "Opt_Selector.lvclass">)  [unwired: 7 in]
          n98 = call-dynamic "Read State.vi"("error in (no error)"=w256, "State Machine in"=w255) -> ("error out"=w257:errorcluster, "State"=w254:i32, "State Machine out"=w258:refnum<class "State Machine.lvclass">)  [unwired: 7 in]
          n99 = Equal To 0?(x=w254) -> (x = 0?=w253:bool)
          n100 = call-dynamic "Write State Machine.vi"("error in (no error)"=w257, "State Machine.lvclass"=w258, "Device in"=w262) -> ("error out"=w263:errorcluster, "Device out"=w261:refnum<class "Opt_Selector.lvclass">)  [unwired: 7 in]
          n101 = call "Write CALW.vi"("error in (no error)"=w263, "Opt_Selector.lvclass"=w261, "Instrument in"=w230) -> ("error out"=w224:errorcluster, "Instrument out"=w225:refnum<class "Instrument.lvclass">)  [unwired: 7 in]
          n102 = call "Read WPSEL.vi"("error in (no error)"=w224, "Instrument in"=w225) -> ("error out"=w247:errorcluster, "Opt_Selector.lvclass"=w246:refnum<class "Opt_Selector.lvclass">, "Instrument out"=w229:refnum<class "Instrument.lvclass">)  [unwired: 7 in]
          n103 = call-dynamic "Read State Machine.vi"("error in (no error)"=w247, "Device in"=w246) -> ("error out"=w250:errorcluster, "State Machine.lvclass"=w251:refnum<class "State Machine.lvclass">, "Device out"=w244:refnum<class "Opt_Selector.lvclass">)  [unwired: 7 in]
          n104 = call-dynamic "Read State.vi"("error in (no error)"=w250, "State Machine in"=w251) -> ("error out"=w249:errorcluster, "State"=w252:i32, "State Machine out"=w248:refnum<class "State Machine.lvclass">)  [unwired: 7 in]
          n105 = Equal To 0?(x=w252) -> (x = 0?=w232:bool)
          n106 = call-dynamic "Write State Machine.vi"("error in (no error)"=w249, "State Machine.lvclass"=w248, "Device in"=w244) -> ("error out"=w243:errorcluster, "Device out"=w245:refnum<class "Opt_Selector.lvclass">)  [unwired: 7 in]
          n107 = call "Write WPSEL.vi"("error in (no error)"=w243, "Opt_Selector.lvclass"=w245, "Instrument in"=w229) -> ("error out"=w222:errorcluster, "Instrument out"=w223:refnum<class "Instrument.lvclass">)  [unwired: 7 in]
          n108 = call "Read WPROT.vi"("error in (no error)"=w222, "Instrument in"=w223) -> ("error out"=w238:errorcluster, "Opt_Selector.lvclass"=w239:refnum<class "Opt_Selector.lvclass">, "Instrument out"=w228:refnum<class "Instrument.lvclass">)  [unwired: 7 in]
          n109 = call-dynamic "Read State Machine.vi"("error in (no error)"=w238, "Device in"=w239) -> ("error out"=w235:errorcluster, "State Machine.lvclass"=w234:refnum<class "State Machine.lvclass">, "Device out"=w241:refnum<class "Opt_Selector.lvclass">)  [unwired: 7 in]
          n110 = call-dynamic "Read State.vi"("error in (no error)"=w235, "State Machine in"=w234) -> ("error out"=w236:errorcluster, "State"=w233:i32, "State Machine out"=w237:refnum<class "State Machine.lvclass">)  [unwired: 7 in]
          n111 = Equal To 0?(x=w233) -> (x = 0?=w231:bool)
          n112 = call-dynamic "Write State Machine.vi"("error in (no error)"=w236, "State Machine.lvclass"=w237, "Device in"=w241) -> ("error out"=w242:errorcluster, "Device out"=w240:refnum<class "Opt_Selector.lvclass">)  [unwired: 7 in]
          n113 = call "Write WPROT.vi"("error in (no error)"=w242, "Opt_Selector.lvclass"=w240, "Instrument in"=w228) -> ("error out"=w220:errorcluster, "Instrument out"=w221:refnum<class "Instrument.lvclass">)  [unwired: 7 in]
          n114 = Compound Arithmetic op=AND(w264, w253, w232, w231) -> (w266:bool)
          n115 = Select(t=u32 0, s=w266, f=w265) -> (s? t:f=w268:u32)
          n116 = call "Write Instrument.lvclass.vi"("error in (no error)"=w220, "Instrument.lvclass"=w221, "S4ACS_GUI in"=w284) -> ("error out"=w281:errorcluster, "S4ACS_GUI out"=w271:refnum<class "S4ACS_GUI.lvclass">)  [unwired: 7 in]
          n117 = Bundle By Name(cluster=w271, "Obs_state"=w268) -> (w270:refnum<class "S4ACS_GUI.lvclass">)
        }
        frame 202 {
          # "Dispara o comando para o dispositivo corrente."
          n118 = call "Read Instrument.lvclass.vi"("error in (no error)"=w303, "S4ACS_GUI in"=w304) -> ("error out"=w309:errorcluster, "Instrument.lvclass"=w310:refnum<class "Instrument.lvclass">, "S4ACS_GUI out"=w306:refnum<class "S4ACS_GUI.lvclass">)  [unwired: 7 in]
          n119 = call "Read CALW.vi"("error in (no error)"=w309, "Instrument in"=w310) -> ("error out"=w296:errorcluster, "Opt_Selector.lvclass"=w295:refnum<class "Opt_Selector.lvclass">, "Instrument out"=w308:refnum<class "Instrument.lvclass">)  [unwired: 7 in]
          n120 = call-dynamic "Read State Machine.vi"("error in (no error)"=w296, "Device in"=w295) -> ("error out"=w299:errorcluster, "State Machine.lvclass"=w301:refnum<class "State Machine.lvclass">, "Device out"=w293:refnum<class "Opt_Selector.lvclass">)  [unwired: 7 in]
          n121 = call "Next State.vi"("error in (no error)"=w299, "New_State"=1, "State Machine in"=w301) -> ("error out"=w298:errorcluster, "State Machine out"=w297:refnum<class "State Machine.lvclass">)  [unwired: 7 in]
          n122 = call-dynamic "Write State Machine.vi"("error in (no error)"=w298, "State Machine.lvclass"=w297, "Device in"=w293) -> ("error out"=w292:errorcluster, "Device out"=w294:refnum<class "Opt_Selector.lvclass">)  [unwired: 7 in]
          n123 = Increment(x=w290) -> (x+1=w289:u32)
          n124 = call "Write CALW.vi"("error in (no error)"=w292, "Opt_Selector.lvclass"=w294, "Instrument in"=w308) -> ("error out"=w305:errorcluster, "Instrument out"=w307:refnum<class "Instrument.lvclass">)  [unwired: 7 in]
          n125 = call "Write Instrument.lvclass.vi"("error in (no error)"=w305, "Instrument.lvclass"=w307, "S4ACS_GUI in"=w306) -> ("error out"=w302:errorcluster, "S4ACS_GUI out"=w291:refnum<class "S4ACS_GUI.lvclass">)  [unwired: 7 in]
          n126 = Bundle By Name(cluster=w291, "Obs_state"=w289) -> (w288:refnum<class "S4ACS_GUI.lvclass">)
        }
        frame 203 {
          # "Espera terminar a execução do comando atual \nantes de ir ao proximo passo da Observação."
          n127 = call "Read Instrument.lvclass.vi"("error in (no error)"=w328, "S4ACS_GUI in"=w329) -> ("error out"=w334:errorcluster, "Instrument.lvclass"=w335:refnum<class "Instrument.lvclass">, "S4ACS_GUI out"=w331:refnum<class "S4ACS_GUI.lvclass">)  [unwired: 7 in]
          n128 = call "Read CALW.vi"("error in (no error)"=w334, "Instrument in"=w335) -> ("error out"=w322:errorcluster, "Opt_Selector.lvclass"=w321:refnum<class "Opt_Selector.lvclass">, "Instrument out"=w333:refnum<class "Instrument.lvclass">)  [unwired: 7 in]
          n129 = call-dynamic "Read State Machine.vi"("error in (no error)"=w322, "Device in"=w321) -> ("error out"=w325:errorcluster, "State Machine.lvclass"=w326:refnum<class "State Machine.lvclass">, "Device out"=w319:refnum<class "Opt_Selector.lvclass">)  [unwired: 7 in]
          n130 = Increment(x=w312) -> (x+1=w311:u32)
          n131 = call-dynamic "Read State.vi"("error in (no error)"=w325, "State Machine in"=w326) -> ("error out"=w324:errorcluster, "State"=w314:i32, "State Machine out"=w323:refnum<class "State Machine.lvclass">)  [unwired: 7 in]
          n132 = Equal To 0?(x=w314) -> (x = 0?=w315:bool)
          n133 = call-dynamic "Write State Machine.vi"("error in (no error)"=w324, "State Machine.lvclass"=w323, "Device in"=w319) -> ("error out"=w318:errorcluster, "Device out"=w320:refnum<class "Opt_Selector.lvclass">)  [unwired: 7 in]
          n134 = call "Write CALW.vi"("error in (no error)"=w318, "Opt_Selector.lvclass"=w320, "Instrument in"=w333) -> ("error out"=w330:errorcluster, "Instrument out"=w332:refnum<class "Instrument.lvclass">)  [unwired: 7 in]
          n135 = Select(t=w311, s=w315, f=w312) -> (s? t:f=w313:u32)
          n136 = call "Write Instrument.lvclass.vi"("error in (no error)"=w330, "Instrument.lvclass"=w332, "S4ACS_GUI in"=w331) -> ("error out"=w327:errorcluster, "S4ACS_GUI out"=w317:refnum<class "S4ACS_GUI.lvclass">)  [unwired: 7 in]
          n137 = Bundle By Name(cluster=w317, "Obs_state"=w313) -> (w316:refnum<class "S4ACS_GUI.lvclass">)
        }
        frame 204 {
          # "Dispara o comando para o dispositivo corrente."
          n138 = call "Read Instrument.lvclass.vi"("error in (no error)"=w351, "S4ACS_GUI in"=w352) -> ("error out"=w357:errorcluster, "Instrument.lvclass"=w358:refnum<class "Instrument.lvclass">, "S4ACS_GUI out"=w354:refnum<class "S4ACS_GUI.lvclass">)  [unwired: 7 in]
          n139 = call "Read WPSEL.vi"("error in (no error)"=w357, "Instrument in"=w358) -> ("error out"=w344:errorcluster, "Opt_Selector.lvclass"=w343:refnum<class "Opt_Selector.lvclass">, "Instrument out"=w356:refnum<class "Instrument.lvclass">)  [unwired: 7 in]
          n140 = call-dynamic "Read State Machine.vi"("error in (no error)"=w344, "Device in"=w343) -> ("error out"=w347:errorcluster, "State Machine.lvclass"=w349:refnum<class "State Machine.lvclass">, "Device out"=w341:refnum<class "Opt_Selector.lvclass">)  [unwired: 7 in]
          n141 = call "Next State.vi"("error in (no error)"=w347, "New_State"=1, "State Machine in"=w349) -> ("error out"=w346:errorcluster, "State Machine out"=w345:refnum<class "State Machine.lvclass">)  [unwired: 7 in]
          n142 = call-dynamic "Write State Machine.vi"("error in (no error)"=w346, "State Machine.lvclass"=w345, "Device in"=w341) -> ("error out"=w340:errorcluster, "Device out"=w342:refnum<class "Opt_Selector.lvclass">)  [unwired: 7 in]
          n143 = Increment(x=w338) -> (x+1=w337:u32)
          n144 = call "Write WPSEL.vi"("error in (no error)"=w340, "Opt_Selector.lvclass"=w342, "Instrument in"=w356) -> ("error out"=w353:errorcluster, "Instrument out"=w355:refnum<class "Instrument.lvclass">)  [unwired: 7 in]
          n145 = call "Write Instrument.lvclass.vi"("error in (no error)"=w353, "Instrument.lvclass"=w355, "S4ACS_GUI in"=w354) -> ("error out"=w350:errorcluster, "S4ACS_GUI out"=w339:refnum<class "S4ACS_GUI.lvclass">)  [unwired: 7 in]
          n146 = Bundle By Name(cluster=w339, "Obs_state"=w337) -> (w336:refnum<class "S4ACS_GUI.lvclass">)
        }
        frame 205 {
          # "Espera terminar a execução do comando atual \nantes de ir ao proximo passo da Observação."
          n147 = call "Read Instrument.lvclass.vi"("error in (no error)"=w376, "S4ACS_GUI in"=w377) -> ("error out"=w382:errorcluster, "Instrument.lvclass"=w383:refnum<class "Instrument.lvclass">, "S4ACS_GUI out"=w379:refnum<class "S4ACS_GUI.lvclass">)  [unwired: 7 in]
          n148 = call "Read WPSEL.vi"("error in (no error)"=w382, "Instrument in"=w383) -> ("error out"=w370:errorcluster, "Opt_Selector.lvclass"=w369:refnum<class "Opt_Selector.lvclass">, "Instrument out"=w381:refnum<class "Instrument.lvclass">)  [unwired: 7 in]
          n149 = call-dynamic "Read State Machine.vi"("error in (no error)"=w370, "Device in"=w369) -> ("error out"=w373:errorcluster, "State Machine.lvclass"=w374:refnum<class "State Machine.lvclass">, "Device out"=w367:refnum<class "Opt_Selector.lvclass">)  [unwired: 7 in]
          n150 = Increment(x=w360) -> (x+1=w359:u32)
          n151 = call-dynamic "Read State.vi"("error in (no error)"=w373, "State Machine in"=w374) -> ("error out"=w372:errorcluster, "State"=w362:i32, "State Machine out"=w371:refnum<class "State Machine.lvclass">)  [unwired: 7 in]
          n152 = Equal To 0?(x=w362) -> (x = 0?=w363:bool)
          n153 = call-dynamic "Write State Machine.vi"("error in (no error)"=w372, "State Machine.lvclass"=w371, "Device in"=w367) -> ("error out"=w366:errorcluster, "Device out"=w368:refnum<class "Opt_Selector.lvclass">)  [unwired: 7 in]
          n154 = call "Write WPSEL.vi"("error in (no error)"=w366, "Opt_Selector.lvclass"=w368, "Instrument in"=w381) -> ("error out"=w378:errorcluster, "Instrument out"=w380:refnum<class "Instrument.lvclass">)  [unwired: 7 in]
          n155 = Select(t=w359, s=w363, f=w360) -> (s? t:f=w361:u32)
          n156 = call "Write Instrument.lvclass.vi"("error in (no error)"=w378, "Instrument.lvclass"=w380, "S4ACS_GUI in"=w379) -> ("error out"=w375:errorcluster, "S4ACS_GUI out"=w365:refnum<class "S4ACS_GUI.lvclass">)  [unwired: 7 in]
          n157 = Bundle By Name(cluster=w365, "Obs_state"=w361) -> (w364:refnum<class "S4ACS_GUI.lvclass">)
        }
        frame 206 {
          # "Dispara o comando para o dispositivo corrente."
          n158 = call "Read Instrument.lvclass.vi"("error in (no error)"=w398, "S4ACS_GUI in"=w399) -> ("error out"=w404:errorcluster, "Instrument.lvclass"=w405:refnum<class "Instrument.lvclass">, "S4ACS_GUI out"=w401:refnum<class "S4ACS_GUI.lvclass">)  [unwired: 7 in]
          n159 = call "Read WPSEL.vi"("error in (no error)"=w404, "Instrument in"=w405) -> ("error out"=w392:errorcluster, "Opt_Selector.lvclass"=w393:refnum<class "Opt_Selector.lvclass">, "Instrument out"=w403:refnum<class "Instrument.lvclass">)  [unwired: 7 in]
          n160 = call "Read target name.vi"("error in (no error)"=w392, "Optics in"=w393) -> ("error out"=w386:errorcluster, "target name"=w391:string, "Optics out"=w385:refnum<class "Opt_Selector.lvclass">)  [unwired: 7 in]
          n161 = Equal?(x=w391, y="OFF") -> (x = y?=w389:bool)
          n162 = Increment(x=w395) -> (x+1=w387:u32)
          n163 = call "Write WPSEL.vi"("error in (no error)"=w386, "Opt_Selector.lvclass"=w385, "Instrument in"=w403) -> ("error out"=w400:errorcluster, "Instrument out"=w402:refnum<class "Instrument.lvclass">)  [unwired: 7 in]
          n164 = Select(t=u32 0, s=w389, f=w387) -> (s? t:f=w384:u32)
          n165 = call "Write Instrument.lvclass.vi"("error in (no error)"=w400, "Instrument.lvclass"=w402, "S4ACS_GUI in"=w401) -> ("error out"=w397:errorcluster, "S4ACS_GUI out"=w396:refnum<class "S4ACS_GUI.lvclass">)  [unwired: 7 in]
          n166 = Bundle By Name(cluster=w396, "Obs_state"=w384) -> (w394:refnum<class "S4ACS_GUI.lvclass">)
        }
        frame 207 {
          # "Dispara o comando para o dispositivo corrente."
          n167 = call "Read Instrument.lvclass.vi"("error in (no error)"=w421, "S4ACS_GUI in"=w422) -> ("error out"=w427:errorcluster, "Instrument.lvclass"=w428:refnum<class "Instrument.lvclass">, "S4ACS_GUI out"=w424:refnum<class "S4ACS_GUI.lvclass">)  [unwired: 7 in]
          n168 = call "Read WPROT.vi"("error in (no error)"=w427, "Instrument in"=w428) -> ("error out"=w414:errorcluster, "Opt_Selector.lvclass"=w413:refnum<class "Opt_Selector.lvclass">, "Instrument out"=w426:refnum<class "Instrument.lvclass">)  [unwired: 7 in]
          n169 = call-dynamic "Read State Machine.vi"("error in (no error)"=w414, "Device in"=w413) -> ("error out"=w417:errorcluster, "State Machine.lvclass"=w419:refnum<class "State Machine.lvclass">, "Device out"=w411:refnum<class "Opt_Selector.lvclass">)  [unwired: 7 in]
          n170 = call "Next State.vi"("error in (no error)"=w417, "New_State"=1, "State Machine in"=w419) -> ("error out"=w416:errorcluster, "State Machine out"=w415:refnum<class "State Machine.lvclass">)  [unwired: 7 in]
          n171 = call-dynamic "Write State Machine.vi"("error in (no error)"=w416, "State Machine.lvclass"=w415, "Device in"=w411) -> ("error out"=w410:errorcluster, "Device out"=w412:refnum<class "Opt_Selector.lvclass">)  [unwired: 7 in]
          n172 = Increment(x=w408) -> (x+1=w407:u32)
          n173 = call "Write WPROT.vi"("error in (no error)"=w410, "Opt_Selector.lvclass"=w412, "Instrument in"=w426) -> ("error out"=w423:errorcluster, "Instrument out"=w425:refnum<class "Instrument.lvclass">)  [unwired: 7 in]
          n174 = call "Write Instrument.lvclass.vi"("error in (no error)"=w423, "Instrument.lvclass"=w425, "S4ACS_GUI in"=w424) -> ("error out"=w420:errorcluster, "S4ACS_GUI out"=w409:refnum<class "S4ACS_GUI.lvclass">)  [unwired: 7 in]
          n175 = Bundle By Name(cluster=w409, "Obs_state"=w407) -> (w406:refnum<class "S4ACS_GUI.lvclass">)
        }
        frame 208 {
          # "Espera terminar a execução do comando atual \nantes de ir ao proximo passo da Observação."
          n176 = call "Read Instrument.lvclass.vi"("error in (no error)"=w446, "S4ACS_GUI in"=w447) -> ("error out"=w452:errorcluster, "Instrument.lvclass"=w453:refnum<class "Instrument.lvclass">, "S4ACS_GUI out"=w449:refnum<class "S4ACS_GUI.lvclass">)  [unwired: 7 in]
          n177 = call "Read WPROT.vi"("error in (no error)"=w452, "Instrument in"=w453) -> ("error out"=w440:errorcluster, "Opt_Selector.lvclass"=w439:refnum<class "Opt_Selector.lvclass">, "Instrument out"=w451:refnum<class "Instrument.lvclass">)  [unwired: 7 in]
          n178 = call-dynamic "Read State Machine.vi"("error in (no error)"=w440, "Device in"=w439) -> ("error out"=w443:errorcluster, "State Machine.lvclass"=w444:refnum<class "State Machine.lvclass">, "Device out"=w437:refnum<class "Opt_Selector.lvclass">)  [unwired: 7 in]
          n179 = call-dynamic "Read State.vi"("error in (no error)"=w443, "State Machine in"=w444) -> ("error out"=w442:errorcluster, "State"=w432:i32, "State Machine out"=w441:refnum<class "State Machine.lvclass">)  [unwired: 7 in]
          n180 = Equal To 0?(x=w432) -> (x = 0?=w433:bool)
          n181 = call-dynamic "Write State Machine.vi"("error in (no error)"=w442, "State Machine.lvclass"=w441, "Device in"=w437) -> ("error out"=w436:errorcluster, "Device out"=w438:refnum<class "Opt_Selector.lvclass">)  [unwired: 7 in]
          n182 = call "Write WPSEL.vi"("error in (no error)"=w436, "Opt_Selector.lvclass"=w438, "Instrument in"=w451) -> ("error out"=w448:errorcluster, "Instrument out"=w450:refnum<class "Instrument.lvclass">)  [unwired: 7 in]
          n183 = Select(t=u32 0, s=w433, f=w430) -> (s? t:f=w431:u32)
          n184 = call "Write Instrument.lvclass.vi"("error in (no error)"=w448, "Instrument.lvclass"=w450, "S4ACS_GUI in"=w449) -> ("error out"=w445:errorcluster, "S4ACS_GUI out"=w435:refnum<class "S4ACS_GUI.lvclass">)  [unwired: 7 in]
          n185 = Bundle By Name(cluster=w435, "Obs_state"=w431) -> (w434:refnum<class "S4ACS_GUI.lvclass">)
        }
        frame 291 {
          n186 = call-dynamic "Read AcquisitionA.vi"("error in (no error)"=w464, "S4ACS_GUI in"=w465) -> ("error out"=w457:errorcluster, "Acquisition.lvclass"=w458:refnum<class "Acquisition.lvclass">, "S4ACS_GUI out"=w467:refnum<class "S4ACS_GUI.lvclass">)  [unwired: 7 in]
          n187 = call "Read connection.vi"("error in (no error)"=w457, "Server in"=w458) -> ("error out"=w456:errorcluster, "connection"=w454:bool, "Server out"=w455:refnum<class "Acquisition.lvclass">)  [unwired: 7 in]
          n188 = case shown="False" w454 {
            tunnel: w455 -> [w473 w493]
            tunnel: w456 -> [w472 w492]
            tunnel: [w473 w490] -> w468
            tunnel: [w472 w489] -> w466
            tunnel: w461 -> [w471 w482]
            tunnel: [w469 w481] -> w460
            frame False {
              n189 = Increment(x=w471) -> (x+1=w470:u32)
              n190 = Increment(x=w470) -> (x+1=w469:u32)
            }
            frame True {
              # "configura o canal,\nmas não dispara\na exposicao."
              n191 = call-dynamic "Read Channel.vi"("error in (no error)"=w492, "Acquisition in"=w493) -> ("error out"=w478:errorcluster, "Channel.lvclass"=w480:refnum<class "Channel.lvclass">, "Acquisition out"=w491:refnum<class "Acquisition.lvclass">)  [unwired: 7 in]
              n192 = call-dynamic "Write expose.vi"("error in (no error)"=w478, "expose"=FALSE, "Channel in"=w480) -> ("error out"=w477:errorcluster, "Channel out"=w479:refnum<class "Channel.lvclass">)  [unwired: 7 in]
              n193 = call-dynamic "Read State Machine.vi"("error in (no error)"=w477, "Device in"=w479) -> ("error out"=w486:errorcluster, "State Machine.lvclass"=w488:refnum<class "State Machine.lvclass">, "Device out"=w484:refnum<class "Channel.lvclass">)  [unwired: 7 in]
              n194 = call "Next State.vi"("error in (no error)"=w486, "New_State"=1, "State Machine in"=w488) -> ("error out"=w474:errorcluster, "State Machine out"=w475:refnum<class "State Machine.lvclass">)  [unwired: 7 in]
              n195 = Increment(x=w482) -> (x+1=w481:u32)
              n196 = call-dynamic "Write State Machine.vi"("error in (no error)"=w474, "State Machine.lvclass"=w475, "Device in"=w484) -> ("error out"=w483:errorcluster, "Device out"=w485:refnum<class "Channel.lvclass">)  [unwired: 7 in]
              n197 = call-dynamic "Write Channel.vi"("error in (no error)"=w483, "Channel.lvclass"=w485, "Acquisition in"=w491) -> ("error out"=w489:errorcluster, "Acquisition out"=w490:refnum<class "Acquisition.lvclass">)  [unwired: 7 in]
            }
          }
          n198 = call-dynamic "Write AcquisitionA.vi"("error in (no error)"=w466, "Acquisition.lvclass"=w468, "S4ACS_GUI in"=w467) -> ("error out"=w463:errorcluster, "S4ACS_GUI out"=w462:refnum<class "S4ACS_GUI.lvclass">)  [unwired: 7 in]
          n199 = Bundle By Name(cluster=w462, "Obs_state"=w460) -> (w459:refnum<class "S4ACS_GUI.lvclass">)
        }
        frame 292 {
          # "Espera terminar a execução do comando atual \nantes de ir ao proximo passo da Observação."
          n200 = call-dynamic "Read AcquisitionA.vi"("error in (no error)"=w511, "S4ACS_GUI in"=w512) -> ("error out"=w517:errorcluster, "Acquisition.lvclass"=w518:refnum<class "Acquisition.lvclass">, "S4ACS_GUI out"=w514:refnum<class "S4ACS_GUI.lvclass">)  [unwired: 7 in]
          n201 = call-dynamic "Read Channel.vi"("error in (no error)"=w517, "Acquisition in"=w518) -> ("error out"=w509:errorcluster, "Channel.lvclass"=w508:refnum<class "Channel.lvclass">, "Acquisition out"=w516:refnum<class "Acquisition.lvclass">)  [unwired: 7 in]
          n202 = call-dynamic "Read State Machine.vi"("error in (no error)"=w509, "Device in"=w508) -> ("error out"=w500:errorcluster, "State Machine.lvclass"=w502:refnum<class "State Machine.lvclass">, "Device out"=w506:refnum<class "Channel.lvclass">)  [unwired: 7 in]
          n203 = call-dynamic "Read State.vi"("error in (no error)"=w500, "State Machine in"=w502) -> ("error out"=w499:errorcluster, "State"=w496:i32, "State Machine out"=w501:refnum<class "State Machine.lvclass">)  [unwired: 7 in]
          n204 = Equal To 0?(x=w496) -> (x = 0?=w498:bool)
          n205 = call-dynamic "Write State Machine.vi"("error in (no error)"=w499, "State Machine.lvclass"=w501, "Device in"=w506) -> ("error out"=w505:errorcluster, "Device out"=w507:refnum<class "Channel.lvclass">)  [unwired: 7 in]
          n206 = call-dynamic "Write Channel.vi"("error in (no error)"=w505, "Channel.lvclass"=w507, "Acquisition in"=w516) -> ("error out"=w513:errorcluster, "Acquisition out"=w515:refnum<class "Acquisition.lvclass">)  [unwired: 7 in]
          n207 = disable-structure shown="Enabled" {
            disable-tunnel: [u32 299 ("t") w520] -> w495
            disable-tunnel: w494 -> [_ w521]
            frame Disabled {
            }
            frame Enabled {
              n208 = Increment(x=w521) -> (x+1=w520:u32)
            }
          }
          n209 = Select(t=w495, s=w498, f=w494) -> (s? t:f=w497:u32)
          n210 = call-dynamic "Write AcquisitionA.vi"("error in (no error)"=w513, "Acquisition.lvclass"=w515, "S4ACS_GUI in"=w514) -> ("error out"=w510:errorcluster, "S4ACS_GUI out"=w504:refnum<class "S4ACS_GUI.lvclass">)  [unwired: 7 in]
          n211 = Bundle By Name(cluster=w504, "Obs_state"=w497) -> (w503:refnum<class "S4ACS_GUI.lvclass">)
        }
        frame 293 {
          n212 = call "Read AcquisitionB.vi"("error in (no error)"=w532, "S4ACS_GUI in"=w533) -> ("error out"=w525:errorcluster, "Acquisition.lvclass"=w526:refnum<class "Acquisition.lvclass">, "S4ACS_GUI out"=w535:refnum<class "S4ACS_GUI.lvclass">)  [unwired: 7 in]
          n213 = call "Read connection.vi"("error in (no error)"=w525, "Server in"=w526) -> ("error out"=w524:errorcluster, "connection"=w522:bool, "Server out"=w523:refnum<class "Acquisition.lvclass">)  [unwired: 7 in]
          n214 = case shown="False" w522 {
            tunnel: w523 -> [w541 w561]
            tunnel: w524 -> [w540 w560]
            tunnel: [w541 w558] -> w536
            tunnel: [w540 w557] -> w534
            tunnel: w529 -> [w539 w550]
            tunnel: [w537 w549] -> w528
            frame False {
              n215 = Increment(x=w539) -> (x+1=w538:u32)
              n216 = Increment(x=w538) -> (x+1=w537:u32)
            }
            frame True {
              # "configura o canal,\nmas não dispara\na exposicao."
              n217 = call-dynamic "Read Channel.vi"("error in (no error)"=w560, "Acquisition in"=w561) -> ("error out"=w546:errorcluster, "Channel.lvclass"=w548:refnum<class "Channel.lvclass">, "Acquisition out"=w559:refnum<class "Acquisition.lvclass">)  [unwired: 7 in]
              n218 = call-dynamic "Write expose.vi"("error in (no error)"=w546, "expose"=FALSE, "Channel in"=w548) -> ("error out"=w545:errorcluster, "Channel out"=w547:refnum<class "Channel.lvclass">)  [unwired: 7 in]
              n219 = call-dynamic "Read State Machine.vi"("error in (no error)"=w545, "Device in"=w547) -> ("error out"=w554:errorcluster, "State Machine.lvclass"=w556:refnum<class "State Machine.lvclass">, "Device out"=w552:refnum<class "Channel.lvclass">)  [unwired: 7 in]
              n220 = call "Next State.vi"("error in (no error)"=w554, "New_State"=1, "State Machine in"=w556) -> ("error out"=w542:errorcluster, "State Machine out"=w543:refnum<class "State Machine.lvclass">)  [unwired: 7 in]
              n221 = Increment(x=w550) -> (x+1=w549:u32)
              n222 = call-dynamic "Write State Machine.vi"("error in (no error)"=w542, "State Machine.lvclass"=w543, "Device in"=w552) -> ("error out"=w551:errorcluster, "Device out"=w553:refnum<class "Channel.lvclass">)  [unwired: 7 in]
              n223 = call-dynamic "Write Channel.vi"("error in (no error)"=w551, "Channel.lvclass"=w553, "Acquisition in"=w559) -> ("error out"=w557:errorcluster, "Acquisition out"=w558:refnum<class "Acquisition.lvclass">)  [unwired: 7 in]
            }
          }
          n224 = call "Write AcquisitionB.vi"("error in (no error)"=w534, "Acquisition.lvclass"=w536, "S4ACS_GUI in"=w535) -> ("error out"=w531:errorcluster, "S4ACS_GUI out"=w530:refnum<class "S4ACS_GUI.lvclass">)  [unwired: 7 in]
          n225 = Bundle By Name(cluster=w530, "Obs_state"=w528) -> (w527:refnum<class "S4ACS_GUI.lvclass">)
        }
        frame 294 {
          # "Espera terminar a execução do comando atual \nantes de ir ao proximo passo da Observação."
          n226 = call "Read AcquisitionB.vi"("error in (no error)"=w579, "S4ACS_GUI in"=w580) -> ("error out"=w585:errorcluster, "Acquisition.lvclass"=w586:refnum<class "Acquisition.lvclass">, "S4ACS_GUI out"=w582:refnum<class "S4ACS_GUI.lvclass">)  [unwired: 7 in]
          n227 = call-dynamic "Read Channel.vi"("error in (no error)"=w585, "Acquisition in"=w586) -> ("error out"=w577:errorcluster, "Channel.lvclass"=w576:refnum<class "Channel.lvclass">, "Acquisition out"=w584:refnum<class "Acquisition.lvclass">)  [unwired: 7 in]
          n228 = call-dynamic "Read State Machine.vi"("error in (no error)"=w577, "Device in"=w576) -> ("error out"=w568:errorcluster, "State Machine.lvclass"=w570:refnum<class "State Machine.lvclass">, "Device out"=w574:refnum<class "Channel.lvclass">)  [unwired: 7 in]
          n229 = call-dynamic "Read State.vi"("error in (no error)"=w568, "State Machine in"=w570) -> ("error out"=w567:errorcluster, "State"=w564:i32, "State Machine out"=w569:refnum<class "State Machine.lvclass">)  [unwired: 7 in]
          n230 = call-dynamic "Write State Machine.vi"("error in (no error)"=w567, "State Machine.lvclass"=w569, "Device in"=w574) -> ("error out"=w573:errorcluster, "Device out"=w575:refnum<class "Channel.lvclass">)  [unwired: 7 in]
          n231 = call-dynamic "Write Channel.vi"("error in (no error)"=w573, "Channel.lvclass"=w575, "Acquisition in"=w584) -> ("error out"=w581:errorcluster, "Acquisition out"=w583:refnum<class "Acquisition.lvclass">)  [unwired: 7 in]
          n232 = Equal To 0?(x=w564) -> (x = 0?=w566:bool)
          n233 = Increment(x=w563) -> (x+1=w562:u32)
          n234 = Select(t=w562, s=w566, f=w563) -> (s? t:f=w565:u32)
          n235 = call "Write AcquisitionB.vi"("error in (no error)"=w581, "Acquisition.lvclass"=w583, "S4ACS_GUI in"=w582) -> ("error out"=w578:errorcluster, "S4ACS_GUI out"=w572:refnum<class "S4ACS_GUI.lvclass">)  [unwired: 7 in]
          n236 = Bundle By Name(cluster=w572, "Obs_state"=w565) -> (w571:refnum<class "S4ACS_GUI.lvclass">)
        }
        frame 295 {
          n237 = call-dynamic "Read AcquisitionC.vi"("error in (no error)"=w597, "S4ACS_GUI in"=w598) -> ("error out"=w589:errorcluster, "Acquisition.lvclass"=w591:refnum<class "Acquisition.lvclass">, "S4ACS_GUI out"=w600:refnum<class "S4ACS_GUI.lvclass">)  [unwired: 7 in]
          n238 = call "Read connection.vi"("error in (no error)"=w589, "Server in"=w591) -> ("error out"=w588:errorcluster, "connection"=w587:bool, "Server out"=w590:refnum<class "Acquisition.lvclass">)  [unwired: 7 in]
          n239 = case shown="True" w587 {
            tunnel: w590 -> [w605 w626]
            tunnel: w588 -> [w606 w625]
            tunnel: [w605 w623] -> w601
            tunnel: [w606 w622] -> w599
            tunnel: w594 -> [w604 w615]
            tunnel: [w602 w614] -> w593
            frame False {
              n240 = Increment(x=w604) -> (x+1=w603:u32)
              n241 = Increment(x=w603) -> (x+1=w602:u32)
            }
            frame True {
              # "configura o canal,\nmas não dispara\na exposicao."
              n242 = call-dynamic "Read Channel.vi"("error in (no error)"=w625, "Acquisition in"=w626) -> ("error out"=w611:errorcluster, "Channel.lvclass"=w613:refnum<class "Channel.lvclass">, "Acquisition out"=w624:refnum<class "Acquisition.lvclass">)  [unwired: 7 in]
              n243 = call-dynamic "Write expose.vi"("error in (no error)"=w611, "expose"=FALSE, "Channel in"=w613) -> ("error out"=w610:errorcluster, "Channel out"=w612:refnum<class "Channel.lvclass">)  [unwired: 7 in]
              n244 = call-dynamic "Read State Machine.vi"("error in (no error)"=w610, "Device in"=w612) -> ("error out"=w619:errorcluster, "State Machine.lvclass"=w621:refnum<class "State Machine.lvclass">, "Device out"=w617:refnum<class "Channel.lvclass">)  [unwired: 7 in]
              n245 = call "Next State.vi"("error in (no error)"=w619, "New_State"=1, "State Machine in"=w621) -> ("error out"=w607:errorcluster, "State Machine out"=w608:refnum<class "State Machine.lvclass">)  [unwired: 7 in]
              n246 = Increment(x=w615) -> (x+1=w614:u32)
              n247 = call-dynamic "Write State Machine.vi"("error in (no error)"=w607, "State Machine.lvclass"=w608, "Device in"=w617) -> ("error out"=w616:errorcluster, "Device out"=w618:refnum<class "Channel.lvclass">)  [unwired: 7 in]
              n248 = call-dynamic "Write Channel.vi"("error in (no error)"=w616, "Channel.lvclass"=w618, "Acquisition in"=w624) -> ("error out"=w622:errorcluster, "Acquisition out"=w623:refnum<class "Acquisition.lvclass">)  [unwired: 7 in]
            }
          }
          n249 = call-dynamic "Write AcquisitionC.vi"("error in (no error)"=w599, "Acquisition.lvclass"=w601, "S4ACS_GUI in"=w600) -> ("error out"=w596:errorcluster, "S4ACS_GUI out"=w595:refnum<class "S4ACS_GUI.lvclass">)  [unwired: 7 in]
          n250 = Bundle By Name(cluster=w595, "Obs_state"=w593) -> (w592:refnum<class "S4ACS_GUI.lvclass">)
        }
        frame 296 {
          # "Espera terminar a execução do comando atual \nantes de ir ao proximo passo da Observação."
          n251 = call-dynamic "Read AcquisitionC.vi"("error in (no error)"=w644, "S4ACS_GUI in"=w645) -> ("error out"=w650:errorcluster, "Acquisition.lvclass"=w651:refnum<class "Acquisition.lvclass">, "S4ACS_GUI out"=w647:refnum<class "S4ACS_GUI.lvclass">)  [unwired: 7 in]
          n252 = call-dynamic "Read Channel.vi"("error in (no error)"=w650, "Acquisition in"=w651) -> ("error out"=w642:errorcluster, "Channel.lvclass"=w641:refnum<class "Channel.lvclass">, "Acquisition out"=w649:refnum<class "Acquisition.lvclass">)  [unwired: 7 in]
          n253 = call-dynamic "Read State Machine.vi"("error in (no error)"=w642, "Device in"=w641) -> ("error out"=w633:errorcluster, "State Machine.lvclass"=w635:refnum<class "State Machine.lvclass">, "Device out"=w639:refnum<class "Channel.lvclass">)  [unwired: 7 in]
          n254 = call-dynamic "Read State.vi"("error in (no error)"=w633, "State Machine in"=w635) -> ("error out"=w632:errorcluster, "State"=w629:i32, "State Machine out"=w634:refnum<class "State Machine.lvclass">)  [unwired: 7 in]
          n255 = Equal To 0?(x=w629) -> (x = 0?=w631:bool)
          n256 = call-dynamic "Write State Machine.vi"("error in (no error)"=w632, "State Machine.lvclass"=w634, "Device in"=w639) -> ("error out"=w638:errorcluster, "Device out"=w640:refnum<class "Channel.lvclass">)  [unwired: 7 in]
          n257 = call-dynamic "Write Channel.vi"("error in (no error)"=w638, "Channel.lvclass"=w640, "Acquisition in"=w649) -> ("error out"=w646:errorcluster, "Acquisition out"=w648:refnum<class "Acquisition.lvclass">)  [unwired: 7 in]
          n258 = Increment(x=w628) -> (x+1=w627:u32)
          n259 = Select(t=w627, s=w631, f=w628) -> (s? t:f=w630:u32)
          n260 = call-dynamic "Write AcquisitionC.vi"("error in (no error)"=w646, "Acquisition.lvclass"=w648, "S4ACS_GUI in"=w647) -> ("error out"=w643:errorcluster, "S4ACS_GUI out"=w637:refnum<class "S4ACS_GUI.lvclass">)  [unwired: 7 in]
          n261 = Bundle By Name(cluster=w637, "Obs_state"=w630) -> (w636:refnum<class "S4ACS_GUI.lvclass">)
        }
        frame 297 {
          # "Dispara o comando para o dispositivo corrente."
          n262 = call-dynamic "Read AcquisitionD.vi"("error in (no error)"=w662, "S4ACS_GUI in"=w663) -> ("error out"=w655:errorcluster, "Acquisition.lvclass"=w656:refnum<class "Acquisition.lvclass">, "S4ACS_GUI out"=w665:refnum<class "S4ACS_GUI.lvclass">)  [unwired: 7 in]
          n263 = call "Read connection.vi"("error in (no error)"=w655, "Server in"=w656) -> ("error out"=w653:errorcluster, "connection"=w652:bool, "Server out"=w654:refnum<class "Acquisition.lvclass">)  [unwired: 7 in]
          n264 = case shown="False" w652 {
            tunnel: w654 -> [w671 w691]
            tunnel: w653 -> [w670 w690]
            tunnel: [w671 w688] -> w666
            tunnel: [w670 w687] -> w664
            tunnel: w659 -> [w669 w680]
            tunnel: [w667 w679] -> w658
            frame False {
              n265 = Increment(x=w669) -> (x+1=w668:u32)
              n266 = Increment(x=w668) -> (x+1=w667:u32)
            }
            frame True {
              # "configura o canal,\nmas não dispara\na exposicao."
              n267 = call-dynamic "Read Channel.vi"("error in (no error)"=w690, "Acquisition in"=w691) -> ("error out"=w676:errorcluster, "Channel.lvclass"=w678:refnum<class "Channel.lvclass">, "Acquisition out"=w689:refnum<class "Acquisition.lvclass">)  [unwired: 7 in]
              n268 = call-dynamic "Write expose.vi"("error in (no error)"=w676, "expose"=FALSE, "Channel in"=w678) -> ("error out"=w675:errorcluster, "Channel out"=w677:refnum<class "Channel.lvclass">)  [unwired: 7 in]
              n269 = call-dynamic "Read State Machine.vi"("error in (no error)"=w675, "Device in"=w677) -> ("error out"=w684:errorcluster, "State Machine.lvclass"=w686:refnum<class "State Machine.lvclass">, "Device out"=w682:refnum<class "Channel.lvclass">)  [unwired: 7 in]
              n270 = call "Next State.vi"("error in (no error)"=w684, "New_State"=1, "State Machine in"=w686) -> ("error out"=w672:errorcluster, "State Machine out"=w673:refnum<class "State Machine.lvclass">)  [unwired: 7 in]
              n271 = Increment(x=w680) -> (x+1=w679:u32)
              n272 = call-dynamic "Write State Machine.vi"("error in (no error)"=w672, "State Machine.lvclass"=w673, "Device in"=w682) -> ("error out"=w681:errorcluster, "Device out"=w683:refnum<class "Channel.lvclass">)  [unwired: 7 in]
              n273 = call-dynamic "Write Channel.vi"("error in (no error)"=w681, "Channel.lvclass"=w683, "Acquisition in"=w689) -> ("error out"=w687:errorcluster, "Acquisition out"=w688:refnum<class "Acquisition.lvclass">)  [unwired: 7 in]
            }
          }
          n274 = call-dynamic "Write AcquisitionD.vi"("error in (no error)"=w664, "Acquisition.lvclass"=w666, "S4ACS_GUI in"=w665) -> ("error out"=w661:errorcluster, "S4ACS_GUI out"=w660:refnum<class "S4ACS_GUI.lvclass">)  [unwired: 7 in]
          n275 = Bundle By Name(cluster=w660, "Obs_state"=w658) -> (w657:refnum<class "S4ACS_GUI.lvclass">)
        }
        frame 298 {
          # "Espera terminar a execução do comando atual \nantes de ir ao proximo passo da Observação."
          n276 = call-dynamic "Read AcquisitionD.vi"("error in (no error)"=w709, "S4ACS_GUI in"=w710) -> ("error out"=w715:errorcluster, "Acquisition.lvclass"=w716:refnum<class "Acquisition.lvclass">, "S4ACS_GUI out"=w712:refnum<class "S4ACS_GUI.lvclass">)  [unwired: 7 in]
          n277 = call-dynamic "Read Channel.vi"("error in (no error)"=w715, "Acquisition in"=w716) -> ("error out"=w707:errorcluster, "Channel.lvclass"=w706:refnum<class "Channel.lvclass">, "Acquisition out"=w714:refnum<class "Acquisition.lvclass">)  [unwired: 7 in]
          n278 = call-dynamic "Read State Machine.vi"("error in (no error)"=w707, "Device in"=w706) -> ("error out"=w698:errorcluster, "State Machine.lvclass"=w700:refnum<class "State Machine.lvclass">, "Device out"=w704:refnum<class "Channel.lvclass">)  [unwired: 7 in]
          n279 = call-dynamic "Read State.vi"("error in (no error)"=w698, "State Machine in"=w700) -> ("error out"=w697:errorcluster, "State"=w694:i32, "State Machine out"=w699:refnum<class "State Machine.lvclass">)  [unwired: 7 in]
          n280 = Equal To 0?(x=w694) -> (x = 0?=w696:bool)
          n281 = call-dynamic "Write State Machine.vi"("error in (no error)"=w697, "State Machine.lvclass"=w699, "Device in"=w704) -> ("error out"=w703:errorcluster, "Device out"=w705:refnum<class "Channel.lvclass">)  [unwired: 7 in]
          n282 = call-dynamic "Write Channel.vi"("error in (no error)"=w703, "Channel.lvclass"=w705, "Acquisition in"=w714) -> ("error out"=w711:errorcluster, "Acquisition out"=w713:refnum<class "Acquisition.lvclass">)  [unwired: 7 in]
          n283 = Increment(x=w693) -> (x+1=w692:u32)
          n284 = Select(t=w692, s=w696, f=w693) -> (s? t:f=w695:u32)
          n285 = call-dynamic "Write AcquisitionD.vi"("error in (no error)"=w711, "Acquisition.lvclass"=w713, "S4ACS_GUI in"=w712) -> ("error out"=w708:errorcluster, "S4ACS_GUI out"=w702:refnum<class "S4ACS_GUI.lvclass">)  [unwired: 7 in]
          n286 = Bundle By Name(cluster=w702, "Obs_state"=w695) -> (w701:refnum<class "S4ACS_GUI.lvclass">)
        }
        frame 299 {
          # "Verifica se é modo fotometria ou polarimetria:\nTrue = polarimetria\nFalse = fotometria"
          n287 = call "Read Instrument.lvclass.vi"("error in (no error)"=w726, "S4ACS_GUI in"=w727) -> ("error out"=w721:errorcluster, "Instrument.lvclass"=w722:refnum<class "Instrument.lvclass">, "S4ACS_GUI out"=w720:refnum<class "S4ACS_GUI.lvclass">)  [unwired: 7 in]
          n288 = call-dynamic "Read mode.vi"("error in (no error)"=w721, "Instrument in"=w722) -> ("error out"=w717:errorcluster, "mode"=w719:bool)  [unwired: 7 in, 1 out]
          n289 = Select(t=u32 301, s=w719, f=u32 321 ("t")) -> (s? t:f=w724:u32)
          n290 = Bundle By Name(cluster=w720, "Obs_state"=w724) -> (w725:refnum<class "S4ACS_GUI.lvclass">)
        }
        frame 301 {
          n291 = call "Read Instrument.lvclass.vi"("error in (no error)"=w762, "S4ACS_GUI in"=w763) -> ("error out"=w766:errorcluster, "Instrument.lvclass"=w767:refnum<class "Instrument.lvclass">, "S4ACS_GUI out"=w764:refnum<class "S4ACS_GUI.lvclass">)  [unwired: 7 in]
          n292 = call "Read WPROT.vi"("error in (no error)"=w766, "Instrument in"=w767) -> ("error out"=w755:errorcluster, "Opt_Selector.lvclass"=w756:refnum<class "Opt_Selector.lvclass">, "Instrument out"=w765:refnum<class "Instrument.lvclass">)  [unwired: 7 in]
          n293 = call-dynamic "getTargetPos.vi"("error in (no error)"=w755, "Opt_Selector in"=w756) -> ("error out"=w754:errorcluster, "Target Pos"=w734:u16, "Opt_Selector out"=w753:refnum<class "Opt_Selector.lvclass">)  [unwired: 7 in]
          n294 = Build Array(-1.0 ("element"), 0.0 ("element"), 22.5 ("element"), 45.0 ("element"), 67.5 ("element"), 90.0 ("element"), 112.5 ("element"), 135.0 ("element"), 157.5 ("element"), 180.0 ("element"), 202.5 ("element"), 225.0 ("element"), 247.5 ("element"), 270.0 ("element"), 292.5 ("element"), 315.0 ("element"), 337.5 ("element")) -> (w746:dbl[])
          n295 = Index Array(array=w746, index=w734) -> (element=w733:dbl)
          n296 = case shown="0, Default" w734 {
            selector: w734 -> [_ w790]
            tunnel: w765 -> [w775 w778]
            tunnel: [w775 w778] -> w729
            tunnel: [w772 w777] -> w728
            tunnel: w759 -> [_ w792]
            tunnel: [u32 311 w791] -> w758
            tunnel: w754 -> [w773 w786]
            tunnel: w753 -> [w774 w785]
            tunnel: w733 -> [_ w780]
            tunnel: [w770 w779] -> w730
            frame 0, Default {
              # "Verifica os ciclos"
              # "Recupera a sequencia anterior para o caso \nde repetição da sequencia (sem precisar clicar \nnas posicoes desejadas novamente)."
              n297 = call-dynamic "Read sequencia_ant.vi"("error in (no error)"=w773, "Opt_Selector in"=w774) -> ("error out"=w769:errorcluster, "sequencia_ant"=w768:u16, "Opt_Selector out"=w771:refnum<class "Opt_Selector.lvclass">)  [unwired: 7 in]
              n298 = call-dynamic "Write sequencia.vi"("error in (no error)"=w769, "sequencia"=w768, "Opt_Selector in"=w771) -> ("error out"=w772:errorcluster, "Opt_Selector out"=w770:refnum<class "Opt_Selector.lvclass">)  [unwired: 7 in]
            }
            frame 1..16 {
              n299 = Number To Decimal String(number=w790) -> (decimal integer string=w789:string)  [unwired: 1 in]
              n300 = Concatenate Strings("WP" ("string"), w789) -> (w787:string)
              n301 = call "Write target name.vi"("error in (no error)"=w786, "target name"=w787, "Optics in"=w785) -> ("error out"=w783:errorcluster, "Optics out"=w784:refnum<class "Opt_Selector.lvclass">)  [unwired: 7 in]
              n302 = call "Write target.vi"("error in (no error)"=w783, "target"=w780, "Optics in"=w784) -> ("error out"=w782:errorcluster, "Optics out"=w781:refnum<class "Opt_Selector.lvclass">)  [unwired: 7 in]
              n303 = call-dynamic "Read State Machine.vi"("error in (no error)"=w782, "Device in"=w781) -> ("error out"=w796:errorcluster, "State Machine.lvclass"=w798:refnum<class "State Machine.lvclass">, "Device out"=w793:refnum<class "Opt_Selector.lvclass">)  [unwired: 7 in]
              n304 = Increment(x=w792) -> (x+1=w791:u32)
              n305 = call "Next State.vi"("error in (no error)"=w796, "New_State"=1, "State Machine in"=w798) -> ("error out"=w795:errorcluster, "State Machine out"=w794:refnum<class "State Machine.lvclass">)  [unwired: 7 in]
              n306 = call-dynamic "Write State Machine.vi"("error in (no error)"=w795, "State Machine.lvclass"=w794, "Device in"=w793) -> ("error out"=w777:errorcluster, "Device out"=w779:refnum<class "Opt_Selector.lvclass">)  [unwired: 7 in]
            }
          }
          n307 = call "Write WPROT.vi"("error in (no error)"=w728, "Opt_Selector.lvclass"=w730, "Instrument in"=w729) -> ("error out"=w732:errorcluster, "Instrument out"=w731:refnum<class "Instrument.lvclass">)  [unwired: 7 in]
          n308 = call "Write Instrument.lvclass.vi"("error in (no error)"=w732, "Instrument.lvclass"=w731, "S4ACS_GUI in"=w764) -> ("error out"=w761:errorcluster, "S4ACS_GUI out"=w760:refnum<class "S4ACS_GUI.lvclass">)  [unwired: 7 in]
          n309 = Bundle By Name(cluster=w760, "Obs_state"=w758) -> (w757:refnum<class "S4ACS_GUI.lvclass">)
        }
        frame 302 {
          # "TESTE: 1 x 20ms = 0.02s de pausa entre \nposições do waveplate."
          # "Espera terminar o movimento para a posição \"target\" do waveplate\nantes de ir para o estado de pausa."
          n310 = call "Read Instrument.lvclass.vi"("error in (no error)"=w819, "S4ACS_GUI in"=w820) -> ("error out"=w825:errorcluster, "Instrument.lvclass"=w826:refnum<class "Instrument.lvclass">, "S4ACS_GUI out"=w822:refnum<class "S4ACS_GUI.lvclass">)  [unwired: 7 in]
          n311 = call "Read WPROT.vi"("error in (no error)"=w825, "Instrument in"=w826) -> ("error out"=w815:errorcluster, "Opt_Selector.lvclass"=w814:refnum<class "Opt_Selector.lvclass">, "Instrument out"=w824:refnum<class "Instrument.lvclass">)  [unwired: 7 in]
          n312 = call-dynamic "Read State Machine.vi"("error in (no error)"=w815, "Device in"=w814) -> ("error out"=w816:errorcluster, "State Machine.lvclass"=w817:refnum<class "State Machine.lvclass">, "Device out"=w812:refnum<class "Opt_Selector.lvclass">)  [unwired: 7 in]
          n313 = Increment(x=w805) -> (x+1=w804:u32)
          n314 = call-dynamic "Read State.vi"("error in (no error)"=w816, "State Machine in"=w817) -> ("error out"=w799:errorcluster, "State"=w807:i32, "State Machine out"=w803:refnum<class "State Machine.lvclass">)  [unwired: 7 in]
          n315 = Equal To 0?(x=w807) -> (x = 0?=w808:bool)
          n316 = call-dynamic "Write Timer.vi"("error in (no error)"=w799, "Timer"=u32 1, "State Machine in"=w803) -> ("error out"=w800:errorcluster, "State Machine out"=w802:refnum<class "State Machine.lvclass">)  [unwired: 7 in]
          n317 = call-dynamic "Write State Machine.vi"("error in (no error)"=w800, "State Machine.lvclass"=w802, "Device in"=w812) -> ("error out"=w811:errorcluster, "Device out"=w813:refnum<class "Opt_Selector.lvclass">)  [unwired: 7 in]
          n318 = call "Write WPROT.vi"("error in (no error)"=w811, "Opt_Selector.lvclass"=w813, "Instrument in"=w824) -> ("error out"=w821:errorcluster, "Instrument out"=w823:refnum<class "Instrument.lvclass">)  [unwired: 7 in]
          n319 = Select(t=w804, s=w808, f=w805) -> (s? t:f=w806:u32)
          n320 = call "Write Instrument.lvclass.vi"("error in (no error)"=w821, "Instrument.lvclass"=w823, "S4ACS_GUI in"=w822) -> ("error out"=w818:errorcluster, "S4ACS_GUI out"=w810:refnum<class "S4ACS_GUI.lvclass">)  [unwired: 7 in]
          n321 = Bundle By Name(cluster=w810, "Obs_state"=w806) -> (w809:refnum<class "S4ACS_GUI.lvclass">)
        }
        frame 303 {
          # "Espera terminar a pausa carregada no Timer"
          n322 = call "Read Instrument.lvclass.vi"("error in (no error)"=w843, "S4ACS_GUI in"=w844) -> ("error out"=w849:errorcluster, "Instrument.lvclass"=w850:refnum<class "Instrument.lvclass">, "S4ACS_GUI out"=w846:refnum<class "S4ACS_GUI.lvclass">)  [unwired: 7 in]
          n323 = call "Read WPROT.vi"("error in (no error)"=w849, "Instrument in"=w850) -> ("error out"=w841:errorcluster, "Opt_Selector.lvclass"=w840:refnum<class "Opt_Selector.lvclass">, "Instrument out"=w848:refnum<class "Instrument.lvclass">)  [unwired: 7 in]
          n324 = call-dynamic "Read State Machine.vi"("error in (no error)"=w841, "Device in"=w840) -> ("error out"=w830:errorcluster, "State Machine.lvclass"=w831:refnum<class "State Machine.lvclass">, "Device out"=w838:refnum<class "Opt_Selector.lvclass">)  [unwired: 7 in]
          n325 = Increment(x=w827) -> (x+1=w832:u32)
          n326 = call "Verify Timer.vi"("error in (no error)"=w830, "State Machine in"=w831) -> ("error out"=w828:errorcluster, "timeout"=w833:bool, "State Machine out"=w829:refnum<class "State Machine.lvclass">)  [unwired: 7 in]
          n327 = call-dynamic "Write State Machine.vi"("error in (no error)"=w828, "State Machine.lvclass"=w829, "Device in"=w838) -> ("error out"=w837:errorcluster, "Device out"=w839:refnum<class "Opt_Selector.lvclass">)  [unwired: 7 in]
          n328 = call "Write WPROT.vi"("error in (no error)"=w837, "Opt_Selector.lvclass"=w839, "Instrument in"=w848) -> ("error out"=w845:errorcluster, "Instrument out"=w847:refnum<class "Instrument.lvclass">)  [unwired: 7 in]
          n329 = call "Write Instrument.lvclass.vi"("error in (no error)"=w845, "Instrument.lvclass"=w847, "S4ACS_GUI in"=w846) -> ("error out"=w842:errorcluster, "S4ACS_GUI out"=w836:refnum<class "S4ACS_GUI.lvclass">)  [unwired: 7 in]
          n330 = Select(t=w832, s=w833, f=w827) -> (s? t:f=w834:u32)
          n331 = Bundle By Name(cluster=w836, "Obs_state"=w834) -> (w835:refnum<class "S4ACS_GUI.lvclass">)
        }
        frame 304 {
          n332 = call-dynamic "Read Sync Box.lvclass.vi"("error in (no error)"=w861, "SPARC4_AC in"=w862) -> ("error out"=w853:errorcluster, "Sync Box.lvclass"=w855:refnum<class "Sync Box.lvclass">, "SPARC4_AC out"=w864:refnum<class "S4ACS_GUI.lvclass">)  [unwired: 7 in]
          n333 = call "Read connection.vi"("error in (no error)"=w853, "Server in"=w855) -> ("error out"=w852:errorcluster, "connection"=w851:bool, "Server out"=w854:refnum<class "Sync Box.lvclass">)  [unwired: 7 in]
          n334 = case shown="False" w851 {
            tunnel: w852 -> [w869 w890]
            tunnel: [w870 w888] -> w865
            tunnel: [w869 w887] -> w863
            tunnel: w858 -> [w868 w878]
            tunnel: [w866 w877] -> w857
            tunnel: w854 -> [w870 w871]
            frame False {
              n335 = Increment(x=w868) -> (x+1=w867:u32)
              n336 = Increment(x=w867) -> (x+1=w866:u32)
            }
            frame True {
              # "configura delays do syncBox"
              n337 = call-dynamic "Read Trigger.lvclass.vi"("error in (no error)"=w890, "Sync Box in"=w871) -> ("error out"=w883:errorcluster, "Trigger.lvclass"=w882:refnum<class "Trigger.lvclass">, "Sync Box out"=w889:refnum<class "Sync Box.lvclass">)  [unwired: 7 in]
              n338 = call-dynamic "Read State Machine.vi"("error in (no error)"=w883, "Device in"=w882) -> ("error out"=w884:errorcluster, "State Machine.lvclass"=w886:refnum<class "State Machine.lvclass">, "Device out"=w880:refnum<class "Trigger.lvclass">)  [unwired: 7 in]
              n339 = call "Next State.vi"("error in (no error)"=w884, "New_State"=10, "State Machine in"=w886) -> ("error out"=w873:errorcluster, "State Machine out"=w875:refnum<class "State Machine.lvclass">)  [unwired: 7 in]
              n340 = Increment(x=w878) -> (x+1=w877:u32)
              n341 = call-dynamic "Write Timer.vi"("error in (no error)"=w873, "Timer"=u32 5, "State Machine in"=w875) -> ("error out"=w872:errorcluster, "State Machine out"=w874:refnum<class "State Machine.lvclass">)  [unwired: 7 in]
              n342 = call-dynamic "Write State Machine.vi"("error in (no error)"=w872, "State Machine.lvclass"=w874, "Device in"=w880) -> ("error out"=w879:errorcluster, "Device out"=w881:refnum<class "Trigger.lvclass">)  [unwired: 7 in]
              n343 = call-dynamic "Write Trigger.lvclass.vi"("error in (no error)"=w879, "Trigger.lvclass"=w881, "Sync Box in"=w889) -> ("error out"=w887:errorcluster, "Sync Box out"=w888:refnum<class "Sync Box.lvclass">)  [unwired: 7 in]
            }
          }
          n344 = call-dynamic "Write Sync Box.lvclass.vi"("error in (no error)"=w863, "Sync Box.lvclass"=w865, "SPARC4_AC in"=w864) -> ("error out"=w860:errorcluster, "SPARC4_AC out"=w859:refnum<class "S4ACS_GUI.lvclass">)  [unwired: 7 in]
          n345 = Bundle By Name(cluster=w859, "Obs_state"=w857) -> (w856:refnum<class "S4ACS_GUI.lvclass">)
        }
        frame 305 {
          # "Espera terminar a execução do comando atual \nantes de ir ao proximo passo da Observação."
          n346 = call-dynamic "Read Sync Box.lvclass.vi"("error in (no error)"=w908, "SPARC4_AC in"=w909) -> ("error out"=w914:errorcluster, "Sync Box.lvclass"=w915:refnum<class "Sync Box.lvclass">, "SPARC4_AC out"=w911:refnum<class "S4ACS_GUI.lvclass">)  [unwired: 7 in]
          n347 = call-dynamic "Read Trigger.lvclass.vi"("error in (no error)"=w914, "Sync Box in"=w915) -> ("error out"=w906:errorcluster, "Trigger.lvclass"=w905:refnum<class "Trigger.lvclass">, "Sync Box out"=w913:refnum<class "Sync Box.lvclass">)  [unwired: 7 in]
          n348 = call-dynamic "Read State Machine.vi"("error in (no error)"=w906, "Device in"=w905) -> ("error out"=w897:errorcluster, "State Machine.lvclass"=w899:refnum<class "State Machine.lvclass">, "Device out"=w903:refnum<class "Trigger.lvclass">)  [unwired: 7 in]
          n349 = call-dynamic "Read State.vi"("error in (no error)"=w897, "State Machine in"=w899) -> ("error out"=w896:errorcluster, "State"=w893:i32, "State Machine out"=w898:refnum<class "State Machine.lvclass">)  [unwired: 7 in]
          n350 = Equal To 0?(x=w893) -> (x = 0?=w895:bool)
          n351 = call-dynamic "Write State Machine.vi"("error in (no error)"=w896, "State Machine.lvclass"=w898, "Device in"=w903) -> ("error out"=w902:errorcluster, "Device out"=w904:refnum<class "Trigger.lvclass">)  [unwired: 7 in]
          n352 = call-dynamic "Write Trigger.lvclass.vi"("error in (no error)"=w902, "Trigger.lvclass"=w904, "Sync Box in"=w913) -> ("error out"=w910:errorcluster, "Sync Box out"=w912:refnum<class "Sync Box.lvclass">)  [unwired: 7 in]
          n353 = Increment(x=w892) -> (x+1=w891:u32)
          n354 = Select(t=w891, s=w895, f=w892) -> (s? t:f=w894:u32)
          n355 = call-dynamic "Write Sync Box.lvclass.vi"("error in (no error)"=w910, "Sync Box.lvclass"=w912, "SPARC4_AC in"=w911) -> ("error out"=w907:errorcluster, "SPARC4_AC out"=w901:refnum<class "S4ACS_GUI.lvclass">)  [unwired: 7 in]
          n356 = Bundle By Name(cluster=w901, "Obs_state"=w894) -> (w900:refnum<class "S4ACS_GUI.lvclass">)
        }
        frame 306 {
          n357 = call-dynamic "Read AcquisitionA.vi"("error in (no error)"=w956, "S4ACS_GUI in"=w957) -> ("error out"=w932:errorcluster, "Acquisition.lvclass"=w935:refnum<class "Acquisition.lvclass">, "S4ACS_GUI out"=w959:refnum<class "S4ACS_GUI.lvclass">)  [unwired: 7 in]
          n358 = call "Read connection.vi"("error in (no error)"=w932, "Server in"=w935) -> ("error out"=w931:errorcluster, "connection"=w933:bool, "Server out"=w934:refnum<class "Acquisition.lvclass">)  [unwired: 7 in]
          n359 = case shown="False" w933 {
            tunnel: w934 -> [w1022 w1040]
            tunnel: w931 -> [w1021 w1039]
            tunnel: [w1022 w1037] -> w960
            tunnel: [w1021 w1036] -> w958
            frame False {
            }
            frame True {
              n360 = call-dynamic "Read Channel.vi"("error in (no error)"=w1039, "Acquisition in"=w1040) -> ("error out"=w1032:errorcluster, "Channel.lvclass"=w1031:refnum<class "Channel.lvclass">, "Acquisition out"=w1038:refnum<class "Acquisition.lvclass">)  [unwired: 7 in]
              n361 = call-dynamic "Read State Machine.vi"("error in (no error)"=w1032, "Device in"=w1031) -> ("error out"=w1033:errorcluster, "State Machine.lvclass"=w1035:refnum<class "State Machine.lvclass">, "Device out"=w1029:refnum<class "Channel.lvclass">)  [unwired: 7 in]
              n362 = call "Next State.vi"("error in (no error)"=w1033, "New_State"=50, "State Machine in"=w1035) -> ("error out"=w1024:errorcluster, "State Machine out"=w1026:refnum<class "State Machine.lvclass">)  [unwired: 7 in]
              n363 = call-dynamic "Write Timer.vi"("error in (no error)"=w1024, "Timer"=u32 2, "State Machine in"=w1026) -> ("error out"=w1023:errorcluster, "State Machine out"=w1025:refnum<class "State Machine.lvclass">)  [unwired: 7 in]
              n364 = call-dynamic "Write State Machine.vi"("error in (no error)"=w1023, "State Machine.lvclass"=w1025, "Device in"=w1029) -> ("error out"=w1028:errorcluster, "Device out"=w1030:refnum<class "Channel.lvclass">)  [unwired: 7 in]
              n365 = call-dynamic "Write Channel.vi"("error in (no error)"=w1028, "Channel.lvclass"=w1030, "Acquisition in"=w1038) -> ("error out"=w1036:errorcluster, "Acquisition out"=w1037:refnum<class "Acquisition.lvclass">)  [unwired: 7 in]
            }
          }
          n366 = call-dynamic "Write AcquisitionA.vi"("error in (no error)"=w958, "Acquisition.lvclass"=w960, "S4ACS_GUI in"=w959) -> ("error out"=w951:errorcluster, "S4ACS_GUI out"=w952:refnum<class "S4ACS_GUI.lvclass">)  [unwired: 7 in]
          n367 = call "Read AcquisitionB.vi"("error in (no error)"=w951, "S4ACS_GUI in"=w952) -> ("error out"=w928:errorcluster, "Acquisition.lvclass"=w930:refnum<class "Acquisition.lvclass">, "S4ACS_GUI out"=w949:refnum<class "S4ACS_GUI.lvclass">)  [unwired: 7 in]
          n368 = call "Read connection.vi"("error in (no error)"=w928, "Server in"=w930) -> ("error out"=w927:errorcluster, "connection"=w926:bool, "Server out"=w929:refnum<class "Acquisition.lvclass">)  [unwired: 7 in]
          n369 = case shown="True" w926 {
            tunnel: w929 -> [w1002 w1020]
            tunnel: w927 -> [w1001 w1019]
            tunnel: [w1002 w1017] -> w950
            tunnel: [w1001 w1016] -> w948
            frame False {
            }
            frame True {
              n370 = call-dynamic "Read Channel.vi"("error in (no error)"=w1019, "Acquisition in"=w1020) -> ("error out"=w1012:errorcluster, "Channel.lvclass"=w1011:refnum<class "Channel.lvclass">, "Acquisition out"=w1018:refnum<class "Acquisition.lvclass">)  [unwired: 7 in]
              n371 = call-dynamic "Read State Machine.vi"("error in (no error)"=w1012, "Device in"=w1011) -> ("error out"=w1013:errorcluster, "State Machine.lvclass"=w1015:refnum<class "State Machine.lvclass">, "Device out"=w1009:refnum<class "Channel.lvclass">)  [unwired: 7 in]
              n372 = call "Next State.vi"("error in (no error)"=w1013, "New_State"=50, "State Machine in"=w1015) -> ("error out"=w1004:errorcluster, "State Machine out"=w1006:refnum<class "State Machine.lvclass">)  [unwired: 7 in]
              n373 = call-dynamic "Write Timer.vi"("error in (no error)"=w1004, "Timer"=u32 2, "State Machine in"=w1006) -> ("error out"=w1003:errorcluster, "State Machine out"=w1005:refnum<class "State Machine.lvclass">)  [unwired: 7 in]
              n374 = call-dynamic "Write State Machine.vi"("error in (no error)"=w1003, "State Machine.lvclass"=w1005, "Device in"=w1009) -> ("error out"=w1008:errorcluster, "Device out"=w1010:refnum<class "Channel.lvclass">)  [unwired: 7 in]
              n375 = call-dynamic "Write Channel.vi"("error in (no error)"=w1008, "Channel.lvclass"=w1010, "Acquisition in"=w1018) -> ("error out"=w1016:errorcluster, "Acquisition out"=w1017:refnum<class "Acquisition.lvclass">)  [unwired: 7 in]
            }
          }
          n376 = call "Write AcquisitionB.vi"("error in (no error)"=w948, "Acquisition.lvclass"=w950, "S4ACS_GUI in"=w949) -> ("error out"=w944:errorcluster, "S4ACS_GUI out"=w943:refnum<class "S4ACS_GUI.lvclass">)  [unwired: 7 in]
          n377 = call-dynamic "Read AcquisitionC.vi"("error in (no error)"=w944, "S4ACS_GUI in"=w943) -> ("error out"=w923:errorcluster, "Acquisition.lvclass"=w925:refnum<class "Acquisition.lvclass">, "S4ACS_GUI out"=w946:refnum<class "S4ACS_GUI.lvclass">)  [unwired: 7 in]
          n378 = call "Read connection.vi"("error in (no error)"=w923, "Server in"=w925) -> ("error out"=w922:errorcluster, "connection"=w921:bool, "Server out"=w924:refnum<class "Acquisition.lvclass">)  [unwired: 7 in]
          n379 = case shown="False" w921 {
            tunnel: [w981 w987] -> w947
            tunnel: [w982 w986] -> w945
            tunnel: w924 -> [w982 w984]
            tunnel: w922 -> [w981 w983]
            frame False {
            }
            frame True {
              n380 = call-dynamic "Read Channel.vi"("error in (no error)"=w983, "Acquisition in"=w984) -> ("error out"=w991:errorcluster, "Channel.lvclass"=w992:refnum<class "Channel.lvclass">, "Acquisition out"=w985:refnum<class "Acquisition.lvclass">)  [unwired: 7 in]
              n381 = call-dynamic "Read State Machine.vi"("error in (no error)"=w991, "Device in"=w992) -> ("error out"=w990:errorcluster, "State Machine.lvclass"=w988:refnum<class "State Machine.lvclass">, "Device out"=w994:refnum<class "Channel.lvclass">)  [unwired: 7 in]
              n382 = call "Next State.vi"("error in (no error)"=w990, "New_State"=50, "State Machine in"=w988) -> ("error out"=w999:errorcluster, "State Machine out"=w997:refnum<class "State Machine.lvclass">)  [unwired: 7 in]
              n383 = call-dynamic "Write Timer.vi"("error in (no error)"=w999, "Timer"=u32 2, "State Machine in"=w997) -> ("error out"=w1000:errorcluster, "State Machine out"=w998:refnum<class "State Machine.lvclass">)  [unwired: 7 in]
              n384 = call-dynamic "Write State Machine.vi"("error in (no error)"=w1000, "State Machine.lvclass"=w998, "Device in"=w994) -> ("error out"=w995:errorcluster, "Device out"=w993:refnum<class "Channel.lvclass">)  [unwired: 7 in]
              n385 = call-dynamic "Write Channel.vi"("error in (no error)"=w995, "Channel.lvclass"=w993, "Acquisition in"=w985) -> ("error out"=w987:errorcluster, "Acquisition out"=w986:refnum<class "Acquisition.lvclass">)  [unwired: 7 in]
            }
          }
          n386 = call-dynamic "Write AcquisitionC.vi"("error in (no error)"=w947, "Acquisition.lvclass"=w945, "S4ACS_GUI in"=w946) -> ("error out"=w941:errorcluster, "S4ACS_GUI out"=w940:refnum<class "S4ACS_GUI.lvclass">)  [unwired: 7 in]
          n387 = call-dynamic "Read AcquisitionD.vi"("error in (no error)"=w941, "S4ACS_GUI in"=w940) -> ("error out"=w918:errorcluster, "Acquisition.lvclass"=w920:refnum<class "Acquisition.lvclass">, "S4ACS_GUI out"=w939:refnum<class "S4ACS_GUI.lvclass">)  [unwired: 7 in]
          n388 = call "Read connection.vi"("error in (no error)"=w918, "Server in"=w920) -> ("error out"=w917:errorcluster, "connection"=w916:bool, "Server out"=w919:refnum<class "Acquisition.lvclass">)  [unwired: 7 in]
          n389 = case shown="False" w916 {
            tunnel: w917 -> [w961 w980]
            tunnel: [w961 w979] -> w942
            tunnel: w919 -> [w962 w965]
            tunnel: [w962 w963] -> w938
            frame False {
            }
            frame True {
              n390 = call-dynamic "Read Channel.vi"("error in (no error)"=w980, "Acquisition in"=w965) -> ("error out"=w975:errorcluster, "Channel.lvclass"=w974:refnum<class "Channel.lvclass">, "Acquisition out"=w964:refnum<class "Acquisition.lvclass">)  [unwired: 7 in]
              n391 = call-dynamic "Read State Machine.vi"("error in (no error)"=w975, "Device in"=w974) -> ("error out"=w976:errorcluster, "State Machine.lvclass"=w978:refnum<class "State Machine.lvclass">, "Device out"=w972:refnum<class "Channel.lvclass">)  [unwired: 7 in]
              n392 = call "Next State.vi"("error in (no error)"=w976, "New_State"=50, "State Machine in"=w978) -> ("error out"=w967:errorcluster, "State Machine out"=w969:refnum<class "State Machine.lvclass">)  [unwired: 7 in]
              n393 = call-dynamic "Write Timer.vi"("error in (no error)"=w967, "Timer"=u32 2, "State Machine in"=w969) -> ("error out"=w966:errorcluster, "State Machine out"=w968:refnum<class "State Machine.lvclass">)  [unwired: 7 in]
              n394 = call-dynamic "Write State Machine.vi"("error in (no error)"=w966, "State Machine.lvclass"=w968, "Device in"=w972) -> ("error out"=w971:errorcluster, "Device out"=w973:refnum<class "Channel.lvclass">)  [unwired: 7 in]
              n395 = call-dynamic "Write Channel.vi"("error in (no error)"=w971, "Channel.lvclass"=w973, "Acquisition in"=w964) -> ("error out"=w979:errorcluster, "Acquisition out"=w963:refnum<class "Acquisition.lvclass">)  [unwired: 7 in]
            }
          }
          n396 = call-dynamic "Write AcquisitionD.vi"("error in (no error)"=w942, "Acquisition.lvclass"=w938, "S4ACS_GUI in"=w939) -> ("error out"=w937:errorcluster, "S4ACS_GUI out"=w936:refnum<class "S4ACS_GUI.lvclass">)  [unwired: 7 in]
          n397 = Increment(x=w955) -> (x+1=w954:u32)
          n398 = Bundle By Name(cluster=w936, "Obs_state"=w954) -> (w953:refnum<class "S4ACS_GUI.lvclass">)
        }
        frame 307 {
          # "Verificar se pode eliminar este estado"
          # "Espera terminar a pausa carregada no Timer"
          n399 = call "Read Instrument.lvclass.vi"("error in (no error)"=w1057, "S4ACS_GUI in"=w1058) -> ("error out"=w1063:errorcluster, "Instrument.lvclass"=w1064:refnum<class "Instrument.lvclass">, "S4ACS_GUI out"=w1060:refnum<class "S4ACS_GUI.lvclass">)  [unwired: 7 in]
          n400 = call "Read WPROT.vi"("error in (no error)"=w1063, "Instrument in"=w1064) -> ("error out"=w1055:errorcluster, "Opt_Selector.lvclass"=w1054:refnum<class "Opt_Selector.lvclass">, "Instrument out"=w1062:refnum<class "Instrument.lvclass">)  [unwired: 7 in]
          n401 = call-dynamic "Read State Machine.vi"("error in (no error)"=w1055, "Device in"=w1054) -> ("error out"=w1044:errorcluster, "State Machine.lvclass"=w1045:refnum<class "State Machine.lvclass">, "Device out"=w1052:refnum<class "Opt_Selector.lvclass">)  [unwired: 7 in]
          n402 = Increment(x=w1041) -> (x+1=w1046:u32)
          n403 = call "Verify Timer.vi"("error in (no error)"=w1044, "State Machine in"=w1045) -> ("error out"=w1042:errorcluster, "timeout"=w1047:bool, "State Machine out"=w1043:refnum<class "State Machine.lvclass">)  [unwired: 7 in]
          n404 = call-dynamic "Write State Machine.vi"("error in (no error)"=w1042, "State Machine.lvclass"=w1043, "Device in"=w1052) -> ("error out"=w1051:errorcluster, "Device out"=w1053:refnum<class "Opt_Selector.lvclass">)  [unwired: 7 in]
          n405 = call "Write WPROT.vi"("error in (no error)"=w1051, "Opt_Selector.lvclass"=w1053, "Instrument in"=w1062) -> ("error out"=w1059:errorcluster, "Instrument out"=w1061:refnum<class "Instrument.lvclass">)  [unwired: 7 in]
          n406 = disable-structure shown="Enabled" {
            disable-tunnel: [w1068 w1069] -> w1048
            disable-tunnel: w1047 -> [w1067 _]
            disable-tunnel: w1046 -> [w1066 w1069]
            disable-tunnel: w1041 -> [w1065 _]
            frame Disabled {
              n407 = Select(t=w1066, s=w1067, f=w1065) -> (s? t:f=w1068:u32)
            }
            frame Enabled {
            }
          }
          n408 = call "Write Instrument.lvclass.vi"("error in (no error)"=w1059, "Instrument.lvclass"=w1061, "S4ACS_GUI in"=w1060) -> ("error out"=w1056:errorcluster, "S4ACS_GUI out"=w1050:refnum<class "S4ACS_GUI.lvclass">)  [unwired: 7 in]
          n409 = Bundle By Name(cluster=w1050, "Obs_state"=w1048) -> (w1049:refnum<class "S4ACS_GUI.lvclass">)
        }
        frame 308 {
          # "Dispara o comando para o dispositivo corrente."
          n410 = call-dynamic "Read Sync Box.lvclass.vi"("error in (no error)"=w1080, "SPARC4_AC in"=w1081) -> ("error out"=w1072:errorcluster, "Sync Box.lvclass"=w1074:refnum<class "Sync Box.lvclass">, "SPARC4_AC out"=w1083:refnum<class "S4ACS_GUI.lvclass">)  [unwired: 7 in]
          n411 = call "Read connection.vi"("error in (no error)"=w1072, "Server in"=w1074) -> ("error out"=w1071:errorcluster, "connection"=w1070:bool, "Server out"=w1073:refnum<class "Sync Box.lvclass">)  [unwired: 7 in]
          n412 = case shown="True" w1070 {
            tunnel: w1071 -> [w1088 w1106]
            tunnel: [w1089 w1104] -> w1084
            tunnel: [w1088 w1103] -> w1082
            tunnel: w1077 -> [w1087 w1094]
            tunnel: [w1085 w1093] -> w1076
            tunnel: w1073 -> [w1089 w1092]
            frame False {
              n413 = Increment(x=w1087) -> (x+1=w1086:u32)
              n414 = Increment(x=w1086) -> (x+1=w1085:u32)
            }
            frame True {
              # "envia comando TRIGGER para o SyncBox"
              n415 = call-dynamic "Read Trigger.lvclass.vi"("error in (no error)"=w1106, "Sync Box in"=w1092) -> ("error out"=w1099:errorcluster, "Trigger.lvclass"=w1098:refnum<class "Trigger.lvclass">, "Sync Box out"=w1105:refnum<class "Sync Box.lvclass">)  [unwired: 7 in]
              n416 = call-dynamic "Read State Machine.vi"("error in (no error)"=w1099, "Device in"=w1098) -> ("error out"=w1100:errorcluster, "State Machine.lvclass"=w1102:refnum<class "State Machine.lvclass">, "Device out"=w1096:refnum<class "Trigger.lvclass">)  [unwired: 7 in]
              n417 = call "Next State.vi"("error in (no error)"=w1100, "New_State"=30, "State Machine in"=w1102) -> ("error out"=w1090:errorcluster, "State Machine out"=w1091:refnum<class "State Machine.lvclass">)  [unwired: 7 in]
              n418 = call-dynamic "Write State Machine.vi"("error in (no error)"=w1090, "State Machine.lvclass"=w1091, "Device in"=w1096) -> ("error out"=w1095:errorcluster, "Device out"=w1097:refnum<class "Trigger.lvclass">)  [unwired: 7 in]
              n419 = Increment(x=w1094) -> (x+1=w1093:u32)
              n420 = call-dynamic "Write Trigger.lvclass.vi"("error in (no error)"=w1095, "Trigger.lvclass"=w1097, "Sync Box in"=w1105) -> ("error out"=w1103:errorcluster, "Sync Box out"=w1104:refnum<class "Sync Box.lvclass">)  [unwired: 7 in]
            }
          }
          n421 = call-dynamic "Write Sync Box.lvclass.vi"("error in (no error)"=w1082, "Sync Box.lvclass"=w1084, "SPARC4_AC in"=w1083) -> ("error out"=w1079:errorcluster, "SPARC4_AC out"=w1078:refnum<class "S4ACS_GUI.lvclass">)  [unwired: 7 in]
          n422 = Bundle By Name(cluster=w1078, "Obs_state"=w1076) -> (w1075:refnum<class "S4ACS_GUI.lvclass">)
        }
        frame 309 {
          # "Espera terminar a execução do comando atual \nantes de ir ao proximo passo da Observação."
          n423 = call-dynamic "Read Sync Box.lvclass.vi"("error in (no error)"=w1124, "SPARC4_AC in"=w1125) -> ("error out"=w1130:errorcluster, "Sync Box.lvclass"=w1131:refnum<class "Sync Box.lvclass">, "SPARC4_AC out"=w1127:refnum<class "S4ACS_GUI.lvclass">)  [unwired: 7 in]
          n424 = call-dynamic "Read Trigger.lvclass.vi"("error in (no error)"=w1130, "Sync Box in"=w1131) -> ("error out"=w1122:errorcluster, "Trigger.lvclass"=w1121:refnum<class "Trigger.lvclass">, "Sync Box out"=w1129:refnum<class "Sync Box.lvclass">)  [unwired: 7 in]
          n425 = call-dynamic "Read State Machine.vi"("error in (no error)"=w1122, "Device in"=w1121) -> ("error out"=w1113:errorcluster, "State Machine.lvclass"=w1115:refnum<class "State Machine.lvclass">, "Device out"=w1119:refnum<class "Trigger.lvclass">)  [unwired: 7 in]
          n426 = call-dynamic "Read State.vi"("error in (no error)"=w1113, "State Machine in"=w1115) -> ("error out"=w1112:errorcluster, "State"=w1109:i32, "State Machine out"=w1114:refnum<class "State Machine.lvclass">)  [unwired: 7 in]
          n427 = Equal To 0?(x=w1109) -> (x = 0?=w1111:bool)
          n428 = call-dynamic "Write State Machine.vi"("error in (no error)"=w1112, "State Machine.lvclass"=w1114, "Device in"=w1119) -> ("error out"=w1118:errorcluster, "Device out"=w1120:refnum<class "Trigger.lvclass">)  [unwired: 7 in]
          n429 = call-dynamic "Write Trigger.lvclass.vi"("error in (no error)"=w1118, "Trigger.lvclass"=w1120, "Sync Box in"=w1129) -> ("error out"=w1126:errorcluster, "Sync Box out"=w1128:refnum<class "Sync Box.lvclass">)  [unwired: 7 in]
          n430 = Increment(x=w1108) -> (x+1=w1107:u32)
          n431 = Select(t=w1107, s=w1111, f=w1108) -> (s? t:f=w1110:u32)
          n432 = call-dynamic "Write Sync Box.lvclass.vi"("error in (no error)"=w1126, "Sync Box.lvclass"=w1128, "SPARC4_AC in"=w1127) -> ("error out"=w1123:errorcluster, "SPARC4_AC out"=w1117:refnum<class "S4ACS_GUI.lvclass">)  [unwired: 7 in]
          n433 = Bundle By Name(cluster=w1117, "Obs_state"=w1110) -> (w1116:refnum<class "S4ACS_GUI.lvclass">)
        }
        frame 310 {
          # "Espera terminar a execução do comando atual \nantes de ir ao proximo passo da Observação."
          n434 = call-dynamic "Read AcquisitionA.vi"("error in (no error)"=w1204, "S4ACS_GUI in"=w1205) -> ("error out"=w1210:errorcluster, "Acquisition.lvclass"=w1211:refnum<class "Acquisition.lvclass">, "S4ACS_GUI out"=w1207:refnum<class "S4ACS_GUI.lvclass">)  [unwired: 7 in]
          n435 = call-dynamic "Read Channel.vi"("error in (no error)"=w1210, "Acquisition in"=w1211) -> ("error out"=w1203:errorcluster, "Channel.lvclass"=w1202:refnum<class "Channel.lvclass">, "Acquisition out"=w1209:refnum<class "Acquisition.lvclass">)  [unwired: 7 in]
          n436 = call-dynamic "Read State Machine.vi"("error in (no error)"=w1203, "Device in"=w1202) -> ("error out"=w1195:errorcluster, "State Machine.lvclass"=w1197:refnum<class "State Machine.lvclass">, "Device out"=w1200:refnum<class "Channel.lvclass">)  [unwired: 7 in]
          n437 = call-dynamic "Read State.vi"("error in (no error)"=w1195, "State Machine in"=w1197) -> ("error out"=w1194:errorcluster, "State"=w1189:i32, "State Machine out"=w1196:refnum<class "State Machine.lvclass">)  [unwired: 7 in]
          n438 = call-dynamic "Write State Machine.vi"("error in (no error)"=w1194, "State Machine.lvclass"=w1196, "Device in"=w1200) -> ("error out"=w1199:errorcluster, "Device out"=w1201:refnum<class "Channel.lvclass">)  [unwired: 7 in]
          n439 = call-dynamic "Write Channel.vi"("error in (no error)"=w1199, "Channel.lvclass"=w1201, "Acquisition in"=w1209) -> ("error out"=w1206:errorcluster, "Acquisition out"=w1208:refnum<class "Acquisition.lvclass">)  [unwired: 7 in]
          n440 = call-dynamic "Write AcquisitionA.vi"("error in (no error)"=w1206, "Acquisition.lvclass"=w1208, "S4ACS_GUI in"=w1207) -> ("error out"=w1190:errorcluster, "S4ACS_GUI out"=w1191:refnum<class "S4ACS_GUI.lvclass">)  [unwired: 7 in]
          n441 = call "Read AcquisitionB.vi"("error in (no error)"=w1190, "S4ACS_GUI in"=w1191) -> ("error out"=w1184:errorcluster, "Acquisition.lvclass"=w1185:refnum<class "Acquisition.lvclass">, "S4ACS_GUI out"=w1181:refnum<class "S4ACS_GUI.lvclass">)  [unwired: 7 in]
          n442 = call-dynamic "Read Channel.vi"("error in (no error)"=w1184, "Acquisition in"=w1185) -> ("error out"=w1179:errorcluster, "Channel.lvclass"=w1178:refnum<class "Channel.lvclass">, "Acquisition out"=w1183:refnum<class "Acquisition.lvclass">)  [unwired: 7 in]
          n443 = call-dynamic "Read State Machine.vi"("error in (no error)"=w1179, "Device in"=w1178) -> ("error out"=w1172:errorcluster, "State Machine.lvclass"=w1174:refnum<class "State Machine.lvclass">, "Device out"=w1176:refnum<class "Channel.lvclass">)  [unwired: 7 in]
          n444 = call-dynamic "Read State.vi"("error in (no error)"=w1172, "State Machine in"=w1174) -> ("error out"=w1171:errorcluster, "State"=w1170:i32, "State Machine out"=w1173:refnum<class "State Machine.lvclass">)  [unwired: 7 in]
          n445 = call-dynamic "Write State Machine.vi"("error in (no error)"=w1171, "State Machine.lvclass"=w1173, "Device in"=w1176) -> ("error out"=w1175:errorcluster, "Device out"=w1177:refnum<class "Channel.lvclass">)  [unwired: 7 in]
          n446 = call-dynamic "Write Channel.vi"("error in (no error)"=w1175, "Channel.lvclass"=w1177, "Acquisition in"=w1183) -> ("error out"=w1180:errorcluster, "Acquisition out"=w1182:refnum<class "Acquisition.lvclass">)  [unwired: 7 in]
          n447 = call "Write AcquisitionB.vi"("error in (no error)"=w1180, "Acquisition.lvclass"=w1182, "S4ACS_GUI in"=w1181) -> ("error out"=w1156:errorcluster, "S4ACS_GUI out"=w1155:refnum<class "S4ACS_GUI.lvclass">)  [unwired: 7 in]
          n448 = call-dynamic "Read AcquisitionC.vi"("error in (no error)"=w1156, "S4ACS_GUI in"=w1155) -> ("error out"=w1158:errorcluster, "Acquisition.lvclass"=w1157:refnum<class "Acquisition.lvclass">, "S4ACS_GUI out"=w1161:refnum<class "S4ACS_GUI.lvclass">)  [unwired: 7 in]
          n449 = call-dynamic "Read Channel.vi"("error in (no error)"=w1158, "Acquisition in"=w1157) -> ("error out"=w1163:errorcluster, "Channel.lvclass"=w1164:refnum<class "Channel.lvclass">, "Acquisition out"=w1159:refnum<class "Acquisition.lvclass">)  [unwired: 7 in]
          n450 = call-dynamic "Read State Machine.vi"("error in (no error)"=w1163, "Device in"=w1164) -> ("error out"=w1153:errorcluster, "State Machine.lvclass"=w1168:refnum<class "State Machine.lvclass">, "Device out"=w1166:refnum<class "Channel.lvclass">)  [unwired: 7 in]
          n451 = call-dynamic "Read State.vi"("error in (no error)"=w1153, "State Machine in"=w1168) -> ("error out"=w1154:errorcluster, "State"=w1152:i32, "State Machine out"=w1169:refnum<class "State Machine.lvclass">)  [unwired: 7 in]
          n452 = call-dynamic "Write State Machine.vi"("error in (no error)"=w1154, "State Machine.lvclass"=w1169, "Device in"=w1166) -> ("error out"=w1167:errorcluster, "Device out"=w1165:refnum<class "Channel.lvclass">)  [unwired: 7 in]
          n453 = call-dynamic "Write Channel.vi"("error in (no error)"=w1167, "Channel.lvclass"=w1165, "Acquisition in"=w1159) -> ("error out"=w1162:errorcluster, "Acquisition out"=w1160:refnum<class "Acquisition.lvclass">)  [unwired: 7 in]
          n454 = call-dynamic "Write AcquisitionC.vi"("error in (no error)"=w1162, "Acquisition.lvclass"=w1160, "S4ACS_GUI in"=w1161) -> ("error out"=w1136:errorcluster, "S4ACS_GUI out"=w1135:refnum<class "S4ACS_GUI.lvclass">)  [unwired: 7 in]
          n455 = call-dynamic "Read AcquisitionD.vi"("error in (no error)"=w1136, "S4ACS_GUI in"=w1135) -> ("error out"=w1150:errorcluster, "Acquisition.lvclass"=w1151:refnum<class "Acquisition.lvclass">, "S4ACS_GUI out"=w1147:refnum<class "S4ACS_GUI.lvclass">)  [unwired: 7 in]
          n456 = call-dynamic "Read Channel.vi"("error in (no error)"=w1150, "Acquisition in"=w1151) -> ("error out"=w1145:errorcluster, "Channel.lvclass"=w1144:refnum<class "Channel.lvclass">, "Acquisition out"=w1149:refnum<class "Acquisition.lvclass">)  [unwired: 7 in]
          n457 = call-dynamic "Read State Machine.vi"("error in (no error)"=w1145, "Device in"=w1144) -> ("error out"=w1138:errorcluster, "State Machine.lvclass"=w1140:refnum<class "State Machine.lvclass">, "Device out"=w1142:refnum<class "Channel.lvclass">)  [unwired: 7 in]
          n458 = call-dynamic "Read State.vi"("error in (no error)"=w1138, "State Machine in"=w1140) -> ("error out"=w1137:errorcluster, "State"=w1134:i32, "State Machine out"=w1139:refnum<class "State Machine.lvclass">)  [unwired: 7 in]
          n459 = call-dynamic "Write State Machine.vi"("error in (no error)"=w1137, "State Machine.lvclass"=w1139, "Device in"=w1142) -> ("error out"=w1141:errorcluster, "Device out"=w1143:refnum<class "Channel.lvclass">)  [unwired: 7 in]
          n460 = call-dynamic "Write Channel.vi"("error in (no error)"=w1141, "Channel.lvclass"=w1143, "Acquisition in"=w1149) -> ("error out"=w1146:errorcluster, "Acquisition out"=w1148:refnum<class "Acquisition.lvclass">)  [unwired: 7 in]
          n461 = call-dynamic "Write AcquisitionD.vi"("error in (no error)"=w1146, "Acquisition.lvclass"=w1148, "S4ACS_GUI in"=w1147) -> ("error out"=w1132:errorcluster, "S4ACS_GUI out"=w1133:refnum<class "S4ACS_GUI.lvclass">)  [unwired: 7 in]
          n462 = Compound Arithmetic op=ADD(w1189, w1170, w1152, w1134) -> (w1188:i32)
          n463 = Equal To 0?(x=w1188) -> (x = 0?=w1193:bool)
          n464 = Select(t=u32 301, s=w1193, f=w1187) -> (s? t:f=w1192:u32)
          n465 = Bundle By Name(cluster=w1133, "Obs_state"=w1192) -> (w1198:refnum<class "S4ACS_GUI.lvclass">)
        }
        frame 311 {
          n466 = call-dynamic "Read ciclos.vi"("error in (no error)"=w1224, "S4ACS_GUI in"=w1225) -> ("error out"=w1213:errorcluster, "ciclos"=w1218:u32, "S4ACS_GUI out"=w1226:refnum<class "S4ACS_GUI.lvclass">)  [unwired: 7 in]
          n467 = Decrement(x=w1218) -> (x-1=w1212:u32)
          n468 = Greater Than 0?(x=w1212) -> (x > 0?=w1219:bool)
          n469 = case shown="False" w1219 {
            selector: w1219 -> [w1228 w1230]
            tunnel: w1212 -> [_ w1229]
            tunnel: [w1228 w1230] -> w1217
            tunnel: [u32 0 w1229] -> w1214
            frame False {
            }
            frame True {
            }
          }
          n470 = Select(t=u32 301, s=w1217, f=u32 0) -> (s? t:f=w1220:u32)
          n471 = call-dynamic "Write ciclos.vi"("error in (no error)"=w1213, "ciclos"=w1214, "S4ACS_GUI in"=w1226) -> ("error out"=w1223:errorcluster, "S4ACS_GUI out"=w1222:refnum<class "S4ACS_GUI.lvclass">)  [unwired: 7 in]
          n472 = Bundle By Name(cluster=w1222, "Obs_state"=w1220) -> (w1221:refnum<class "S4ACS_GUI.lvclass">)
        }
        frame 321 {
          n473 = call-dynamic "Read Sync Box.lvclass.vi"("error in (no error)"=w1241, "SPARC4_AC in"=w1242) -> ("error out"=w1236:errorcluster, "Sync Box.lvclass"=w1237:refnum<class "Sync Box.lvclass">, "SPARC4_AC out"=w1244:refnum<class "S4ACS_GUI.lvclass">)  [unwired: 7 in]
          n474 = call "Read connection.vi"("error in (no error)"=w1236, "Server in"=w1237) -> ("error out"=w1235:errorcluster, "connection"=w1234:bool, "Server out"=w1233:refnum<class "Sync Box.lvclass">)  [unwired: 7 in]
          n475 = case shown="False" w1234 {
            tunnel: [w1250 w1269] -> w1245
            tunnel: [w1249 w1268] -> w1243
            tunnel: w1235 -> [w1249 w1254]
            tunnel: w1233 -> [w1250 w1253]
            tunnel: w1232 -> [w1248 w1252]
            tunnel: [w1246 w1251] -> w1231
            frame False {
              # "SyncBox desconectado. Desvia do estado de espera para configuração do SyncBox...."
              n476 = Increment(x=w1248) -> (x+1=w1247:u32)
              n477 = Increment(x=w1247) -> (x+1=w1246:u32)
            }
            frame True {
              # "Configura os \"delays\" do syncBox"
              n478 = call-dynamic "Read Trigger.lvclass.vi"("error in (no error)"=w1254, "Sync Box in"=w1253) -> ("error out"=w1264:errorcluster, "Trigger.lvclass"=w1263:refnum<class "Trigger.lvclass">, "Sync Box out"=w1270:refnum<class "Sync Box.lvclass">)  [unwired: 7 in]
              n479 = call-dynamic "Read State Machine.vi"("error in (no error)"=w1264, "Device in"=w1263) -> ("error out"=w1265:errorcluster, "State Machine.lvclass"=w1267:refnum<class "State Machine.lvclass">, "Device out"=w1261:refnum<class "Trigger.lvclass">)  [unwired: 7 in]
              n480 = call "Next State.vi"("error in (no error)"=w1265, "New_State"=10, "State Machine in"=w1267) -> ("error out"=w1256:errorcluster, "State Machine out"=w1258:refnum<class "State Machine.lvclass">)  [unwired: 7 in]
              n481 = call-dynamic "Write Timer.vi"("error in (no error)"=w1256, "Timer"=u32 5, "State Machine in"=w1258) -> ("error out"=w1255:errorcluster, "State Machine out"=w1257:refnum<class "State Machine.lvclass">)  [unwired: 7 in]
              n482 = call-dynamic "Write State Machine.vi"("error in (no error)"=w1255, "State Machine.lvclass"=w1257, "Device in"=w1261) -> ("error out"=w1260:errorcluster, "Device out"=w1262:refnum<class "Trigger.lvclass">)  [unwired: 7 in]
              n483 = Increment(x=w1252) -> (x+1=w1251:u32)
              n484 = call-dynamic "Write Trigger.lvclass.vi"("error in (no error)"=w1260, "Trigger.lvclass"=w1262, "Sync Box in"=w1270) -> ("error out"=w1268:errorcluster, "Sync Box out"=w1269:refnum<class "Sync Box.lvclass">)  [unwired: 7 in]
            }
          }
          n485 = call-dynamic "Write Sync Box.lvclass.vi"("error in (no error)"=w1243, "Sync Box.lvclass"=w1245, "SPARC4_AC in"=w1244) -> ("error out"=w1240:errorcluster, "SPARC4_AC out"=w1239:refnum<class "S4ACS_GUI.lvclass">)  [unwired: 7 in]
          n486 = Bundle By Name(cluster=w1239, "Obs_state"=w1231) -> (w1238:refnum<class "S4ACS_GUI.lvclass">)
        }
        frame 322 {
          # "Espera terminar a execução do comando atual \nantes de ir ao proximo passo da Observação."
          n487 = call-dynamic "Read Sync Box.lvclass.vi"("error in (no error)"=w1288, "SPARC4_AC in"=w1289) -> ("error out"=w1294:errorcluster, "Sync Box.lvclass"=w1295:refnum<class "Sync Box.lvclass">, "SPARC4_AC out"=w1291:refnum<class "S4ACS_GUI.lvclass">)  [unwired: 7 in]
          n488 = call-dynamic "Read Trigger.lvclass.vi"("error in (no error)"=w1294, "Sync Box in"=w1295) -> ("error out"=w1286:errorcluster, "Trigger.lvclass"=w1285:refnum<class "Trigger.lvclass">, "Sync Box out"=w1293:refnum<class "Sync Box.lvclass">)  [unwired: 7 in]
          n489 = call-dynamic "Read State Machine.vi"("error in (no error)"=w1286, "Device in"=w1285) -> ("error out"=w1277:errorcluster, "State Machine.lvclass"=w1279:refnum<class "State Machine.lvclass">, "Device out"=w1283:refnum<class "Trigger.lvclass">)  [unwired: 7 in]
          n490 = call-dynamic "Read State.vi"("error in (no error)"=w1277, "State Machine in"=w1279) -> ("error out"=w1276:errorcluster, "State"=w1273:i32, "State Machine out"=w1278:refnum<class "State Machine.lvclass">)  [unwired: 7 in]
          n491 = Equal To 0?(x=w1273) -> (x = 0?=w1275:bool)
          n492 = call-dynamic "Write State Machine.vi"("error in (no error)"=w1276, "State Machine.lvclass"=w1278, "Device in"=w1283) -> ("error out"=w1282:errorcluster, "Device out"=w1284:refnum<class "Trigger.lvclass">)  [unwired: 7 in]
          n493 = call-dynamic "Write Trigger.lvclass.vi"("error in (no error)"=w1282, "Trigger.lvclass"=w1284, "Sync Box in"=w1293) -> ("error out"=w1290:errorcluster, "Sync Box out"=w1292:refnum<class "Sync Box.lvclass">)  [unwired: 7 in]
          n494 = Increment(x=w1272) -> (x+1=w1271:u32)
          n495 = Select(t=w1271, s=w1275, f=w1272) -> (s? t:f=w1274:u32)
          n496 = call-dynamic "Write Sync Box.lvclass.vi"("error in (no error)"=w1290, "Sync Box.lvclass"=w1292, "SPARC4_AC in"=w1291) -> ("error out"=w1287:errorcluster, "SPARC4_AC out"=w1281:refnum<class "S4ACS_GUI.lvclass">)  [unwired: 7 in]
          n497 = Bundle By Name(cluster=w1281, "Obs_state"=w1274) -> (w1280:refnum<class "S4ACS_GUI.lvclass">)
        }
        frame 323 {
          n498 = call-dynamic "Read AcquisitionA.vi"("error in (no error)"=w1298, "S4ACS_GUI in"=w1299) -> ("error out"=w1316:errorcluster, "Acquisition.lvclass"=w1319:refnum<class "Acquisition.lvclass">, "S4ACS_GUI out"=w1336:refnum<class "S4ACS_GUI.lvclass">)  [unwired: 7 in]
          n499 = call "Read connection.vi"("error in (no error)"=w1316, "Server in"=w1319) -> ("error out"=w1315:errorcluster, "connection"=w1317:bool, "Server out"=w1318:refnum<class "Acquisition.lvclass">)  [unwired: 7 in]
          n500 = case shown="False" w1317 {
            tunnel: w1318 -> [w1402 w1420]
            tunnel: w1315 -> [w1401 w1419]
            tunnel: [w1402 w1417] -> w1337
            tunnel: [w1401 w1416] -> w1335
            frame False {
            }
            frame True {
              n501 = call-dynamic "Read Channel.vi"("error in (no error)"=w1419, "Acquisition in"=w1420) -> ("error out"=w1412:errorcluster, "Channel.lvclass"=w1411:refnum<class "Channel.lvclass">, "Acquisition out"=w1418:refnum<class "Acquisition.lvclass">)  [unwired: 7 in]
              n502 = call-dynamic "Read State Machine.vi"("error in (no error)"=w1412, "Device in"=w1411) -> ("error out"=w1413:errorcluster, "State Machine.lvclass"=w1415:refnum<class "State Machine.lvclass">, "Device out"=w1409:refnum<class "Channel.lvclass">)  [unwired: 7 in]
              n503 = call "Next State.vi"("error in (no error)"=w1413, "New_State"=50, "State Machine in"=w1415) -> ("error out"=w1404:errorcluster, "State Machine out"=w1406:refnum<class "State Machine.lvclass">)  [unwired: 7 in]
              n504 = call-dynamic "Write Timer.vi"("error in (no error)"=w1404, "Timer"=u32 2, "State Machine in"=w1406) -> ("error out"=w1403:errorcluster, "State Machine out"=w1405:refnum<class "State Machine.lvclass">)  [unwired: 7 in]
              n505 = call-dynamic "Write State Machine.vi"("error in (no error)"=w1403, "State Machine.lvclass"=w1405, "Device in"=w1409) -> ("error out"=w1408:errorcluster, "Device out"=w1410:refnum<class "Channel.lvclass">)  [unwired: 7 in]
              n506 = call-dynamic "Write Channel.vi"("error in (no error)"=w1408, "Channel.lvclass"=w1410, "Acquisition in"=w1418) -> ("error out"=w1416:errorcluster, "Acquisition out"=w1417:refnum<class "Acquisition.lvclass">)  [unwired: 7 in]
            }
          }
          n507 = call-dynamic "Write AcquisitionA.vi"("error in (no error)"=w1335, "Acquisition.lvclass"=w1337, "S4ACS_GUI in"=w1336) -> ("error out"=w1333:errorcluster, "S4ACS_GUI out"=w1334:refnum<class "S4ACS_GUI.lvclass">)  [unwired: 7 in]
          n508 = call "Read AcquisitionB.vi"("error in (no error)"=w1333, "S4ACS_GUI in"=w1334) -> ("error out"=w1312:errorcluster, "Acquisition.lvclass"=w1314:refnum<class "Acquisition.lvclass">, "S4ACS_GUI out"=w1331:refnum<class "S4ACS_GUI.lvclass">)  [unwired: 7 in]
          n509 = call "Read connection.vi"("error in (no error)"=w1312, "Server in"=w1314) -> ("error out"=w1311:errorcluster, "connection"=w1310:bool, "Server out"=w1313:refnum<class "Acquisition.lvclass">)  [unwired: 7 in]
          n510 = case shown="True" w1310 {
            tunnel: w1313 -> [w1382 w1400]
            tunnel: w1311 -> [w1381 w1399]
            tunnel: [w1382 w1397] -> w1332
            tunnel: [w1381 w1396] -> w1330
            frame False {
            }
            frame True {
              n511 = call-dynamic "Read Channel.vi"("error in (no error)"=w1399, "Acquisition in"=w1400) -> ("error out"=w1392:errorcluster, "Channel.lvclass"=w1391:refnum<class "Channel.lvclass">, "Acquisition out"=w1398:refnum<class "Acquisition.lvclass">)  [unwired: 7 in]
              n512 = call-dynamic "Read State Machine.vi"("error in (no error)"=w1392, "Device in"=w1391) -> ("error out"=w1393:errorcluster, "State Machine.lvclass"=w1395:refnum<class "State Machine.lvclass">, "Device out"=w1389:refnum<class "Channel.lvclass">)  [unwired: 7 in]
              n513 = call "Next State.vi"("error in (no error)"=w1393, "New_State"=50, "State Machine in"=w1395) -> ("error out"=w1384:errorcluster, "State Machine out"=w1386:refnum<class "State Machine.lvclass">)  [unwired: 7 in]
              n514 = call-dynamic "Write Timer.vi"("error in (no error)"=w1384, "Timer"=u32 2, "State Machine in"=w1386) -> ("error out"=w1383:errorcluster, "State Machine out"=w1385:refnum<class "State Machine.lvclass">)  [unwired: 7 in]
              n515 = call-dynamic "Write State Machine.vi"("error in (no error)"=w1383, "State Machine.lvclass"=w1385, "Device in"=w1389) -> ("error out"=w1388:errorcluster, "Device out"=w1390:refnum<class "Channel.lvclass">)  [unwired: 7 in]
              n516 = call-dynamic "Write Channel.vi"("error in (no error)"=w1388, "Channel.lvclass"=w1390, "Acquisition in"=w1398) -> ("error out"=w1396:errorcluster, "Acquisition out"=w1397:refnum<class "Acquisition.lvclass">)  [unwired: 7 in]
            }
          }
          n517 = call "Write AcquisitionB.vi"("error in (no error)"=w1330, "Acquisition.lvclass"=w1332, "S4ACS_GUI in"=w1331) -> ("error out"=w1326:errorcluster, "S4ACS_GUI out"=w1325:refnum<class "S4ACS_GUI.lvclass">)  [unwired: 7 in]
          n518 = call-dynamic "Read AcquisitionC.vi"("error in (no error)"=w1326, "S4ACS_GUI in"=w1325) -> ("error out"=w1307:errorcluster, "Acquisition.lvclass"=w1309:refnum<class "Acquisition.lvclass">, "S4ACS_GUI out"=w1328:refnum<class "S4ACS_GUI.lvclass">)  [unwired: 7 in]
          n519 = call "Read connection.vi"("error in (no error)"=w1307, "Server in"=w1309) -> ("error out"=w1306:errorcluster, "connection"=w1305:bool, "Server out"=w1308:refnum<class "Acquisition.lvclass">)  [unwired: 7 in]
          n520 = case shown="False" w1305 {
            tunnel: [w1361 w1367] -> w1329
            tunnel: [w1362 w1366] -> w1327
            tunnel: w1308 -> [w1362 w1364]
            tunnel: w1306 -> [w1361 w1363]
            frame False {
            }
            frame True {
              n521 = call-dynamic "Read Channel.vi"("error in (no error)"=w1363, "Acquisition in"=w1364) -> ("error out"=w1371:errorcluster, "Channel.lvclass"=w1372:refnum<class "Channel.lvclass">, "Acquisition out"=w1365:refnum<class "Acquisition.lvclass">)  [unwired: 7 in]
              n522 = call-dynamic "Read State Machine.vi"("error in (no error)"=w1371, "Device in"=w1372) -> ("error out"=w1370:errorcluster, "State Machine.lvclass"=w1368:refnum<class "State Machine.lvclass">, "Device out"=w1374:refnum<class "Channel.lvclass">)  [unwired: 7 in]
              n523 = call "Next State.vi"("error in (no error)"=w1370, "New_State"=50, "State Machine in"=w1368) -> ("error out"=w1379:errorcluster, "State Machine out"=w1377:refnum<class "State Machine.lvclass">)  [unwired: 7 in]
              n524 = call-dynamic "Write Timer.vi"("error in (no error)"=w1379, "Timer"=u32 2, "State Machine in"=w1377) -> ("error out"=w1380:errorcluster, "State Machine out"=w1378:refnum<class "State Machine.lvclass">)  [unwired: 7 in]
              n525 = call-dynamic "Write State Machine.vi"("error in (no error)"=w1380, "State Machine.lvclass"=w1378, "Device in"=w1374) -> ("error out"=w1375:errorcluster, "Device out"=w1373:refnum<class "Channel.lvclass">)  [unwired: 7 in]
              n526 = call-dynamic "Write Channel.vi"("error in (no error)"=w1375, "Channel.lvclass"=w1373, "Acquisition in"=w1365) -> ("error out"=w1367:errorcluster, "Acquisition out"=w1366:refnum<class "Acquisition.lvclass">)  [unwired: 7 in]
            }
          }
          n527 = call-dynamic "Write AcquisitionC.vi"("error in (no error)"=w1329, "Acquisition.lvclass"=w1327, "S4ACS_GUI in"=w1328) -> ("error out"=w1323:errorcluster, "S4ACS_GUI out"=w1322:refnum<class "S4ACS_GUI.lvclass">)  [unwired: 7 in]
          n528 = call-dynamic "Read AcquisitionD.vi"("error in (no error)"=w1323, "S4ACS_GUI in"=w1322) -> ("error out"=w1302:errorcluster, "Acquisition.lvclass"=w1304:refnum<class "Acquisition.lvclass">, "S4ACS_GUI out"=w1321:refnum<class "S4ACS_GUI.lvclass">)  [unwired: 7 in]
          n529 = call "Read connection.vi"("error in (no error)"=w1302, "Server in"=w1304) -> ("error out"=w1301:errorcluster, "connection"=w1300:bool, "Server out"=w1303:refnum<class "Acquisition.lvclass">)  [unwired: 7 in]
          n530 = case shown="False" w1300 {
            tunnel: w1301 -> [w1341 w1360]
            tunnel: [w1341 w1359] -> w1324
            tunnel: w1303 -> [w1342 w1345]
            tunnel: [w1342 w1343] -> w1320
            frame False {
            }
            frame True {
              n531 = call-dynamic "Read Channel.vi"("error in (no error)"=w1360, "Acquisition in"=w1345) -> ("error out"=w1355:errorcluster, "Channel.lvclass"=w1354:refnum<class "Channel.lvclass">, "Acquisition out"=w1344:refnum<class "Acquisition.lvclass">)  [unwired: 7 in]
              n532 = call-dynamic "Read State Machine.vi"("error in (no error)"=w1355, "Device in"=w1354) -> ("error out"=w1356:errorcluster, "State Machine.lvclass"=w1358:refnum<class "State Machine.lvclass">, "Device out"=w1352:refnum<class "Channel.lvclass">)  [unwired: 7 in]
              n533 = call "Next State.vi"("error in (no error)"=w1356, "New_State"=50, "State Machine in"=w1358) -> ("error out"=w1347:errorcluster, "State Machine out"=w1349:refnum<class "State Machine.lvclass">)  [unwired: 7 in]
              n534 = call-dynamic "Write Timer.vi"("error in (no error)"=w1347, "Timer"=u32 2, "State Machine in"=w1349) -> ("error out"=w1346:errorcluster, "State Machine out"=w1348:refnum<class "State Machine.lvclass">)  [unwired: 7 in]
              n535 = call-dynamic "Write State Machine.vi"("error in (no error)"=w1346, "State Machine.lvclass"=w1348, "Device in"=w1352) -> ("error out"=w1351:errorcluster, "Device out"=w1353:refnum<class "Channel.lvclass">)  [unwired: 7 in]
              n536 = call-dynamic "Write Channel.vi"("error in (no error)"=w1351, "Channel.lvclass"=w1353, "Acquisition in"=w1344) -> ("error out"=w1359:errorcluster, "Acquisition out"=w1343:refnum<class "Acquisition.lvclass">)  [unwired: 7 in]
            }
          }
          n537 = call-dynamic "Write AcquisitionD.vi"("error in (no error)"=w1324, "Acquisition.lvclass"=w1320, "S4ACS_GUI in"=w1321) -> ("error out"=w1296:errorcluster, "S4ACS_GUI out"=w1297:refnum<class "S4ACS_GUI.lvclass">)  [unwired: 7 in]
          n538 = Increment(x=w1340) -> (x+1=w1339:u32)
          n539 = Bundle By Name(cluster=w1297, "Obs_state"=w1339) -> (w1338:refnum<class "S4ACS_GUI.lvclass">)
        }
        frame 324 {
          n540 = call-dynamic "Read Sync Box.lvclass.vi"("error in (no error)"=w1431, "SPARC4_AC in"=w1432) -> ("error out"=w1424:errorcluster, "Sync Box.lvclass"=w1427:refnum<class "Sync Box.lvclass">, "SPARC4_AC out"=w1434:refnum<class "S4ACS_GUI.lvclass">)  [unwired: 7 in]
          n541 = call "Read connection.vi"("error in (no error)"=w1424, "Server in"=w1427) -> ("error out"=w1425:errorcluster, "connection"=w1423:bool, "Server out"=w1426:refnum<class "Sync Box.lvclass">)  [unwired: 7 in]
          n542 = case shown="True" w1423 {
            tunnel: w1425 -> [w1439 w1457]
            tunnel: [w1440 w1455] -> w1435
            tunnel: [w1439 w1454] -> w1433
            tunnel: w1426 -> [w1440 w1445]
            tunnel: w1422 -> [w1438 w1442]
            tunnel: [w1436 w1441] -> w1421
            frame False {
              # "SyncBox desconectado. Desvia do estado de disparo do SyncBox...."
              n543 = Increment(x=w1438) -> (x+1=w1437:u32)
              n544 = Increment(x=w1437) -> (x+1=w1436:u32)
            }
            frame True {
              # "Envia comando TRIGGER para o SyncBox"
              n545 = call-dynamic "Read Trigger.lvclass.vi"("error in (no error)"=w1457, "Sync Box in"=w1445) -> ("error out"=w1450:errorcluster, "Trigger.lvclass"=w1449:refnum<class "Trigger.lvclass">, "Sync Box out"=w1456:refnum<class "Sync Box.lvclass">)  [unwired: 7 in]
              n546 = call-dynamic "Read State Machine.vi"("error in (no error)"=w1450, "Device in"=w1449) -> ("error out"=w1451:errorcluster, "State Machine.lvclass"=w1453:refnum<class "State Machine.lvclass">, "Device out"=w1447:refnum<class "Trigger.lvclass">)  [unwired: 7 in]
              n547 = call "Next State.vi"("error in (no error)"=w1451, "New_State"=30, "State Machine in"=w1453) -> ("error out"=w1443:errorcluster, "State Machine out"=w1444:refnum<class "State Machine.lvclass">)  [unwired: 7 in]
              n548 = Increment(x=w1442) -> (x+1=w1441:u32)
              n549 = call-dynamic "Write State Machine.vi"("error in (no error)"=w1443, "State Machine.lvclass"=w1444, "Device in"=w1447) -> ("error out"=w1446:errorcluster, "Device out"=w1448:refnum<class "Trigger.lvclass">)  [unwired: 7 in]
              n550 = call-dynamic "Write Trigger.lvclass.vi"("error in (no error)"=w1446, "Trigger.lvclass"=w1448, "Sync Box in"=w1456) -> ("error out"=w1454:errorcluster, "Sync Box out"=w1455:refnum<class "Sync Box.lvclass">)  [unwired: 7 in]
            }
          }
          n551 = call-dynamic "Write Sync Box.lvclass.vi"("error in (no error)"=w1433, "Sync Box.lvclass"=w1435, "SPARC4_AC in"=w1434) -> ("error out"=w1430:errorcluster, "SPARC4_AC out"=w1429:refnum<class "S4ACS_GUI.lvclass">)  [unwired: 7 in]
          n552 = Bundle By Name(cluster=w1429, "Obs_state"=w1421) -> (w1428:refnum<class "S4ACS_GUI.lvclass">)
        }
        frame 325 {
          # "Espera terminar a execução do comando atual \nantes de ir ao proximo passo da Observação."
          n553 = call-dynamic "Read Sync Box.lvclass.vi"("error in (no error)"=w1475, "SPARC4_AC in"=w1476) -> ("error out"=w1481:errorcluster, "Sync Box.lvclass"=w1482:refnum<class "Sync Box.lvclass">, "SPARC4_AC out"=w1478:refnum<class "S4ACS_GUI.lvclass">)  [unwired: 7 in]
          n554 = call-dynamic "Read Trigger.lvclass.vi"("error in (no error)"=w1481, "Sync Box in"=w1482) -> ("error out"=w1473:errorcluster, "Trigger.lvclass"=w1472:refnum<class "Trigger.lvclass">, "Sync Box out"=w1480:refnum<class "Sync Box.lvclass">)  [unwired: 7 in]
          n555 = call-dynamic "Read State Machine.vi"("error in (no error)"=w1473, "Device in"=w1472) -> ("error out"=w1464:errorcluster, "State Machine.lvclass"=w1466:refnum<class "State Machine.lvclass">, "Device out"=w1470:refnum<class "Trigger.lvclass">)  [unwired: 7 in]
          n556 = call-dynamic "Read State.vi"("error in (no error)"=w1464, "State Machine in"=w1466) -> ("error out"=w1463:errorcluster, "State"=w1460:i32, "State Machine out"=w1465:refnum<class "State Machine.lvclass">)  [unwired: 7 in]
          n557 = Equal To 0?(x=w1460) -> (x = 0?=w1462:bool)
          n558 = call-dynamic "Write State Machine.vi"("error in (no error)"=w1463, "State Machine.lvclass"=w1465, "Device in"=w1470) -> ("error out"=w1469:errorcluster, "Device out"=w1471:refnum<class "Trigger.lvclass">)  [unwired: 7 in]
          n559 = call-dynamic "Write Trigger.lvclass.vi"("error in (no error)"=w1469, "Trigger.lvclass"=w1471, "Sync Box in"=w1480) -> ("error out"=w1477:errorcluster, "Sync Box out"=w1479:refnum<class "Sync Box.lvclass">)  [unwired: 7 in]
          n560 = Increment(x=w1459) -> (x+1=w1458:u32)
          n561 = Select(t=w1458, s=w1462, f=w1459) -> (s? t:f=w1461:u32)
          n562 = call-dynamic "Write Sync Box.lvclass.vi"("error in (no error)"=w1477, "Sync Box.lvclass"=w1479, "SPARC4_AC in"=w1478) -> ("error out"=w1474:errorcluster, "SPARC4_AC out"=w1468:refnum<class "S4ACS_GUI.lvclass">)  [unwired: 7 in]
          n563 = Bundle By Name(cluster=w1468, "Obs_state"=w1461) -> (w1467:refnum<class "S4ACS_GUI.lvclass">)
        }
        frame 326 {
          # "Espera terminar a execução do comando atual \nantes de ir ao proximo passo da Observação."
          n564 = call-dynamic "Read AcquisitionA.vi"("error in (no error)"=w1555, "S4ACS_GUI in"=w1556) -> ("error out"=w1561:errorcluster, "Acquisition.lvclass"=w1562:refnum<class "Acquisition.lvclass">, "S4ACS_GUI out"=w1558:refnum<class "S4ACS_GUI.lvclass">)  [unwired: 7 in]
          n565 = call-dynamic "Read Channel.vi"("error in (no error)"=w1561, "Acquisition in"=w1562) -> ("error out"=w1554:errorcluster, "Channel.lvclass"=w1553:refnum<class "Channel.lvclass">, "Acquisition out"=w1560:refnum<class "Acquisition.lvclass">)  [unwired: 7 in]
          n566 = call-dynamic "Read State Machine.vi"("error in (no error)"=w1554, "Device in"=w1553) -> ("error out"=w1546:errorcluster, "State Machine.lvclass"=w1548:refnum<class "State Machine.lvclass">, "Device out"=w1551:refnum<class "Channel.lvclass">)  [unwired: 7 in]
          n567 = call-dynamic "Read State.vi"("error in (no error)"=w1546, "State Machine in"=w1548) -> ("error out"=w1545:errorcluster, "State"=w1528:i32, "State Machine out"=w1547:refnum<class "State Machine.lvclass">)  [unwired: 7 in]
          n568 = call-dynamic "Write State Machine.vi"("error in (no error)"=w1545, "State Machine.lvclass"=w1547, "Device in"=w1551) -> ("error out"=w1550:errorcluster, "Device out"=w1552:refnum<class "Channel.lvclass">)  [unwired: 7 in]
          n569 = call-dynamic "Write Channel.vi"("error in (no error)"=w1550, "Channel.lvclass"=w1552, "Acquisition in"=w1560) -> ("error out"=w1557:errorcluster, "Acquisition out"=w1559:refnum<class "Acquisition.lvclass">)  [unwired: 7 in]
          n570 = call-dynamic "Write AcquisitionA.vi"("error in (no error)"=w1557, "Acquisition.lvclass"=w1559, "S4ACS_GUI in"=w1558) -> ("error out"=w1524:errorcluster, "S4ACS_GUI out"=w1523:refnum<class "S4ACS_GUI.lvclass">)  [unwired: 7 in]
          n571 = call "Read AcquisitionB.vi"("error in (no error)"=w1524, "S4ACS_GUI in"=w1523) -> ("error out"=w1531:errorcluster, "Acquisition.lvclass"=w1530:refnum<class "Acquisition.lvclass">, "S4ACS_GUI out"=w1529:refnum<class "S4ACS_GUI.lvclass">)  [unwired: 7 in]
          n572 = call-dynamic "Read Channel.vi"("error in (no error)"=w1531, "Acquisition in"=w1530) -> ("error out"=w1533:errorcluster, "Channel.lvclass"=w1534:refnum<class "Channel.lvclass">, "Acquisition out"=w1532:refnum<class "Acquisition.lvclass">)  [unwired: 7 in]
          n573 = call-dynamic "Read State Machine.vi"("error in (no error)"=w1533, "Device in"=w1534) -> ("error out"=w1540:errorcluster, "State Machine.lvclass"=w1538:refnum<class "State Machine.lvclass">, "Device out"=w1536:refnum<class "Channel.lvclass">)  [unwired: 7 in]
          n574 = call-dynamic "Read State.vi"("error in (no error)"=w1540, "State Machine in"=w1538) -> ("error out"=w1541:errorcluster, "State"=w1527:i32, "State Machine out"=w1539:refnum<class "State Machine.lvclass">)  [unwired: 7 in]
          n575 = call-dynamic "Write State Machine.vi"("error in (no error)"=w1541, "State Machine.lvclass"=w1539, "Device in"=w1536) -> ("error out"=w1537:errorcluster, "Device out"=w1535:refnum<class "Channel.lvclass">)  [unwired: 7 in]
          n576 = call-dynamic "Write Channel.vi"("error in (no error)"=w1537, "Channel.lvclass"=w1535, "Acquisition in"=w1532) -> ("error out"=w1522:errorcluster, "Acquisition out"=w1521:refnum<class "Acquisition.lvclass">)  [unwired: 7 in]
          n577 = call "Write AcquisitionB.vi"("error in (no error)"=w1522, "Acquisition.lvclass"=w1521, "S4ACS_GUI in"=w1529) -> ("error out"=w1490:errorcluster, "S4ACS_GUI out"=w1489:refnum<class "S4ACS_GUI.lvclass">)  [unwired: 7 in]
          n578 = call-dynamic "Read AcquisitionC.vi"("error in (no error)"=w1490, "S4ACS_GUI in"=w1489) -> ("error out"=w1492:errorcluster, "Acquisition.lvclass"=w1491:refnum<class "Acquisition.lvclass">, "S4ACS_GUI out"=w1495:refnum<class "S4ACS_GUI.lvclass">)  [unwired: 7 in]
          n579 = call-dynamic "Read Channel.vi"("error in (no error)"=w1492, "Acquisition in"=w1491) -> ("error out"=w1497:errorcluster, "Channel.lvclass"=w1498:refnum<class "Channel.lvclass">, "Acquisition out"=w1493:refnum<class "Acquisition.lvclass">)  [unwired: 7 in]
          n580 = call-dynamic "Read State Machine.vi"("error in (no error)"=w1497, "Device in"=w1498) -> ("error out"=w1504:errorcluster, "State Machine.lvclass"=w1502:refnum<class "State Machine.lvclass">, "Device out"=w1500:refnum<class "Channel.lvclass">)  [unwired: 7 in]
          n581 = call-dynamic "Read State.vi"("error in (no error)"=w1504, "State Machine in"=w1502) -> ("error out"=w1505:errorcluster, "State"=w1484:i32, "State Machine out"=w1503:refnum<class "State Machine.lvclass">)  [unwired: 7 in]
          n582 = call-dynamic "Write State Machine.vi"("error in (no error)"=w1505, "State Machine.lvclass"=w1503, "Device in"=w1500) -> ("error out"=w1501:errorcluster, "Device out"=w1499:refnum<class "Channel.lvclass">)  [unwired: 7 in]
          n583 = call-dynamic "Write Channel.vi"("error in (no error)"=w1501, "Channel.lvclass"=w1499, "Acquisition in"=w1493) -> ("error out"=w1496:errorcluster, "Acquisition out"=w1494:refnum<class "Acquisition.lvclass">)  [unwired: 7 in]
          n584 = call-dynamic "Write AcquisitionC.vi"("error in (no error)"=w1496, "Acquisition.lvclass"=w1494, "S4ACS_GUI in"=w1495) -> ("error out"=w1487:errorcluster, "S4ACS_GUI out"=w1488:refnum<class "S4ACS_GUI.lvclass">)  [unwired: 7 in]
          n585 = call-dynamic "Read AcquisitionD.vi"("error in (no error)"=w1487, "S4ACS_GUI in"=w1488) -> ("error out"=w1516:errorcluster, "Acquisition.lvclass"=w1517:refnum<class "Acquisition.lvclass">, "S4ACS_GUI out"=w1518:refnum<class "S4ACS_GUI.lvclass">)  [unwired: 7 in]
          n586 = call-dynamic "Read Channel.vi"("error in (no error)"=w1516, "Acquisition in"=w1517) -> ("error out"=w1514:errorcluster, "Channel.lvclass"=w1513:refnum<class "Channel.lvclass">, "Acquisition out"=w1515:refnum<class "Acquisition.lvclass">)  [unwired: 7 in]
          n587 = call-dynamic "Read State Machine.vi"("error in (no error)"=w1514, "Device in"=w1513) -> ("error out"=w1507:errorcluster, "State Machine.lvclass"=w1509:refnum<class "State Machine.lvclass">, "Device out"=w1511:refnum<class "Channel.lvclass">)  [unwired: 7 in]
          n588 = call-dynamic "Read State.vi"("error in (no error)"=w1507, "State Machine in"=w1509) -> ("error out"=w1506:errorcluster, "State"=w1483:i32, "State Machine out"=w1508:refnum<class "State Machine.lvclass">)  [unwired: 7 in]
          n589 = call-dynamic "Write State Machine.vi"("error in (no error)"=w1506, "State Machine.lvclass"=w1508, "Device in"=w1511) -> ("error out"=w1510:errorcluster, "Device out"=w1512:refnum<class "Channel.lvclass">)  [unwired: 7 in]
          n590 = call-dynamic "Write Channel.vi"("error in (no error)"=w1510, "Channel.lvclass"=w1512, "Acquisition in"=w1515) -> ("error out"=w1519:errorcluster, "Acquisition out"=w1520:refnum<class "Acquisition.lvclass">)  [unwired: 7 in]
          n591 = call-dynamic "Write AcquisitionD.vi"("error in (no error)"=w1519, "Acquisition.lvclass"=w1520, "S4ACS_GUI in"=w1518) -> ("error out"=w1485:errorcluster, "S4ACS_GUI out"=w1486:refnum<class "S4ACS_GUI.lvclass">)  [unwired: 7 in]
          n592 = Compound Arithmetic op=ADD(w1528, w1527, w1484, w1483) -> (w1525:i32)
          n593 = Equal To 0?(x=w1525) -> (x = 0?=w1526:bool)
          n594 = Increment(x=w1543) -> (x+1=w1542:u32)
          n595 = Select(t=w1542, s=w1526, f=w1543) -> (s? t:f=w1544:u32)
          n596 = Bundle By Name(cluster=w1486, "Obs_state"=w1544) -> (w1549:refnum<class "S4ACS_GUI.lvclass">)
        }
        frame 327 {
          n597 = call-dynamic "Read ciclos.vi"("error in (no error)"=w1575, "S4ACS_GUI in"=w1576) -> ("error out"=w1564:errorcluster, "ciclos"=w1569:u32, "S4ACS_GUI out"=w1577:refnum<class "S4ACS_GUI.lvclass">)  [unwired: 7 in]
          n598 = Decrement(x=w1569) -> (x-1=w1563:u32)
          n599 = Greater Than 0?(x=w1563) -> (x > 0?=w1570:bool)
          n600 = case shown="True" w1570 {
            selector: w1570 -> [w1579 w1581]
            tunnel: w1563 -> [_ w1580]
            tunnel: [w1579 w1581] -> w1568
            tunnel: [u32 0 w1580] -> w1565
            frame False {
            }
            frame True {
            }
          }
          n601 = Select(t=u32 321, s=w1568, f=u32 0) -> (s? t:f=w1571:u32)
          n602 = call-dynamic "Write ciclos.vi"("error in (no error)"=w1564, "ciclos"=w1565, "S4ACS_GUI in"=w1577) -> ("error out"=w1574:errorcluster, "S4ACS_GUI out"=w1573:refnum<class "S4ACS_GUI.lvclass">)  [unwired: 7 in]
          n603 = Bundle By Name(cluster=w1573, "Obs_state"=w1571) -> (w1572:refnum<class "S4ACS_GUI.lvclass">)
        }
        frame 400 {
          # "Estado de \"Pause\": fica parado aqui até o botão START seja pressionado."
        }
      }
    }
    frame Error {
    }
  }
  "error out" <- w3
  "S4ACS_GUI out" <- w1
